vi "Signal Generator.vi"() -> ()   [LabVIEW 2020]
uses:
  <userlib>/ArtDAQ/_SubVI/ArtDAQ_CreateAOVoltageChan.vi
  <vilib>/Utility/xml.llb/Read From XML File(string).vi
  <vilib>/Utility/config.llb/Read Key (I32).vi
  <vilib>/Utility/config.llb/Read Key (Double).vi
  <vilib>/Utility/config.llb/Read Key (Boolean).vi
  <userlib>/ArtDAQ/_SubVI/ArtDAQ_Write Analog DBL NChan NSamp.vi
  <userlib>/ArtDAQ/_SubVI/ArtDAQ_CfgSampClkTiming.vi
  <vilib>/Utility/xml.llb/Write to XML File(string).vi
  <vilib>/Utility/config.llb/Write Key (U32).vi
  <vilib>/Utility/config.llb/Write Key (Double).vi
  <vilib>/Utility/config.llb/Write Key (Boolean).vi
  <vilib>/measure/NI_MABase.lvlib
  <vilib>/Utility/config.llb/NI_LVConfig.lvlib
  Parameter Settings.vi
panel:
  out "车型数组":string[](array[string])
  in  "Stop":bool
  in  "AO3 Channel":u32(ring)=4 items=["Hall Channel 1", "Hall Channel 2", "ME Channel 1", "ME Channel 2", "ME Channel 3", "ME Channel 4"]
  in  "AO2 Channel":u32(ring)=3 items=["Hall Channel 1", "Hall Channel 1", "ME Channel 1", "ME Channel 2", "ME Channel 3", "ME Channel 4"]
  in  "AO1 Channel":u32(ring)=2 items=["Hall Channel 1", "Hall Channel 2", "ME Channel 1", "ME Channel 2", "ME Channel 3", "ME Channel 4"]
  in  "AO0 Channel":u32(ring) items=["Hall Channel 1", "Hall Channel 2", "ME Channel 1", "ME Channel 2", "ME Channel 3", "ME Channel 3"]
  out "转速表":dbl(knob) scale=0.0..3000.0
  in  "Speed FM":dbl(knob)=583.5936811226446 caption="转速调频" scale=50.0..1000.0
  in  "Brand":u32(ring)=2 items=["Carter", "Keith", "Hitachi", "Kobelco", "Volvo", "Modern", "Komatsu", "Sumitomo"]
  in  "Vehicle Signal":u32(ring) items=["58+2 sinusoid SK140-8", "Hino J05E new 4 cylinder", "Hino J08E new 6 cylinder"]
  out "ME Channel 4":waveform(dbl)(graph)
  out "ME Channel 3":dynamicdata(graph)
  out "ME Channel 2":waveform(dbl)(graph)
  out "ME Channel 1":dynamicdata(graph)
  out "Hall Channel 2":waveform(dbl)(graph)
  out "Hall Channel 1":T1
  out "数组大小":i32
  out "品牌":string
  out "品牌数组":string[](array[string])
  in  "error":errorcluster caption="错误输入（无错误）"
  in  "字符串数组类型":string[](array[string])
  out "数值合法":bool
  out "凸轮轴参数":T2
  out "0凸轮轴信号类型":u32
  out "0凸轮轴电压幅值":dbl format="%#.1f"
  out "0信号个数":dbl=7.0 caption="信号个数" format="%#.1f"
  out "0凸轮轴个数":dbl=1.0 caption="凸轮轴个数" format="%#.1f"
  out "0凸轮轴是否取反":bool
  out "0凸轮轴周期":dbl=3.0 caption="凸轮轴周期" format="%#.1f"
  out "0起始偏移":dbl=3.0 caption="凸轮轴周期" format="%#.1f"
  out "0插齿间隔":dbl=3.0 caption="凸轮轴周期" format="%#.1f"
  out "0间隔齿数":dbl=3.0 caption="凸轮轴周期" format="%#.1f"
  out "曲轴参数":T3
  out "0曲轴轴信号类型":u32
  out "0曲轴电压幅值":dbl format="%#.1f"
  out "0总齿数":dbl=7.0 caption="信号个数" format="%#.1f"
  out "0曲轴个数":dbl=1.0 caption="凸轮轴个数" format="%#.1f"
  out "0曲轴是否取反":bool
  out "0缺齿数":dbl=3.0 caption="凸轮轴周期" format="%#.1f"
  out "0曲轴圈数":dbl=3.0 caption="凸轮轴周期" format="%#.1f"
  out "0缺齿偏移":dbl=3.0 caption="凸轮轴周期" format="%#.1f"
  out "品牌车型数组":string[](array[string])
  out "凸轮轴信号类型":u16(ring) items=["磁电式", "霍尔式", "无曲轴"]
  out "每通道采样数":i32
  in  "采样速率":dbl=50000.0
  in  "物理通道":string(combo)="Dev1/ao0:3"
  out "错误输出":errorcluster
  out "曲轴圈数信号":dynamicdata(graph)
  out "1缺齿偏移":dbl=4.0
  out "缺齿偏移":dbl=8.2 format="%_2f"
  out "长平组信号正弦":dynamicdata(graph)
  out "间隔长平+正弦信号":dynamicdata(graph)
  out "曲轴组合波形":waveform(dbl)(graph)
  out "1曲轴圈数":dbl=4.0
  out "曲轴圈数":dbl=8.2
  out "长平组信号":dynamicdata(graph)
  out "间隔长平+凸信号":dynamicdata(graph)
  out "间隔齿数":dbl=3.0
  out "1间隔齿数":dbl=3.0 caption="凸轮轴周期"
  out "1插齿间隔":dbl=3.0 caption="凸轮轴周期"
  out "1起始偏移":dbl=3.0 caption="凸轮轴周期"
  out "插齿间隔":dbl=8.2
  out "起始偏移":dbl=8.2
  out "车型数组大小":i32
  in  "error":errorcluster caption="错误输入（无错误）"
  in  "字符串数组类型":string[](array[string])
  out "凸轮轴周期·":dbl=8.2 caption="凸轮轴周期"
  out "凸轮轴个数":dbl=8.2
  out "曲轴个数":dbl=8.2
  out "信号个数":dbl=8.2
  out "凸轮轴是否取反":bool
  out "凸轮轴电压幅值":dbl=8.2 format="%0.2p"
  out "曲轴是否取反":bool
  out "曲轴信号类型":u16(ring) items=["磁电式", "霍尔式", "无曲轴"]
  out "缺齿数":dbl=4.0
  out "总齿数":dbl=60.0
  out "曲轴电压幅值":dbl=8.2 format="%0.2p"
  out "1凸轮轴周期·":dbl=3.0 caption="凸轮轴周期"
  out "1凸轮轴是否取反":bool
  out "1凸轮轴个数":dbl=1.0 caption="凸轮轴个数"
  out "1信号个数":dbl=7.0 caption="信号个数"
  out "1凸轮轴电压幅值":dbl=5.0 caption="凸轮轴电压幅值" format="%0.2p"
  out "1凸轮轴信号类型":u16(ring)=1 items=["磁电式", "霍尔式", "无凸轮轴"]
  out "1缺齿数":dbl=4.0
  out "1总齿数":dbl=60.0
  out "1曲轴个数":dbl=2.0 caption="曲轴个数"
  out "1曲轴是否取反":bool
  out "1曲轴电压幅值":dbl=18.0 caption="曲轴电压幅值" format="%0.2p"
  out "1曲轴信号类型":u16(ring) items=["磁电式", "霍尔式", "无曲轴"]
  out "1波形图":waveform(dbl)(graph)
  out "起始偏移（方波）":dbl
  out "起始偏移（正弦）":dbl=0.5
  out "中短平+2正弦":dynamicdata(graph)
  out "长平+1正弦":dynamicdata(graph)
  out "长水平线数量（正弦）":dbl
  out "一个正弦波形图":waveform(dbl)(graph)
  out "起始水平线个数（正弦）":dbl
  out "起始平+1正弦":dynamicdata(graph)
  out "6波形图":waveform(dbl)(graph)
  out "5波形图":waveform(dbl)(graph)
  out "起始水平线个数（方波）":dbl
  out "长平+1凸":dynamicdata(graph)
  out "长水平线数量（方波）":dbl
  out "曲轴":dynamicdata(graph)
  out "曲轴方波缺齿波形图":dynamicdata(graph)
  out "曲轴方波偏移量":dbl=8.2 format="%0.2p"
  out "曲轴方波波形图":waveform(dbl)(graph)
  out "中、短平+2凸":dynamicdata(graph)
  out "起始平+1凸":dynamicdata(graph)
  out "一个凸起波形图":dynamicdata(graph)
  out "曲轴正弦偏移量":dbl caption="偏移量" format="%0.2p"
  out "曲轴正弦波形图":waveform(dbl)(graph)
  out "完\n整\n缺\n齿\n波":waveform(dbl)(graph)
  out "未\n翻\n转\n半\n缺\n齿":dynamicdata(graph)
  out "圆\n弧\n+\n水\n平":dynamicdata(graph)
  out "半\n缺\n齿\n水\n平\n线":waveform(dbl)(graph)
  out "圆\n弧":waveform(dbl)(graph)
  out "t0":timestamp
  out "x轴取点间隔":dbl
  out "循环次数":i32
  out "圆弧点数":dbl=33.0 format="%0.2p"
  out "dt":dbl
  out "圆半径":dbl=2.48 format="%0.2p"
  out "部分\n正弦\n波形图":waveform(dbl)(graph)
  in  "波形发生率Fs":dbl=50000.0
types:
  T1 = typedef "控件 1.ctl" = waveform(dbl)
  T2 = cluster{"0凸轮轴信号类型":u32, "0凸轮轴电压幅值":dbl, "0信号个数":dbl, "0凸轮轴个数":dbl, "0凸轮轴是否取反":bool, "0凸轮轴周期":dbl, "0起始偏移":dbl, "0插齿间隔":dbl, "0间隔齿数":dbl}
  T3 = cluster{"0曲轴轴信号类型":u32, "0曲轴电压幅值":dbl, "0总齿数":dbl, "0曲轴个数":dbl, "0曲轴是否取反":bool, "0却齿数":dbl, "0曲轴圈数":dbl, "0缺齿偏移":dbl}
  T4 = typedef "NI_LVConfig.lvlib/Config Data RefNum.ctl" = refnum<k1>
  T5 = cluster{"0曲轴轴信号类型":u32, "0曲轴电压幅值":dbl, "0总齿数":dbl, "0曲轴个数":dbl, "0曲轴是否取反":bool, "0缺齿数":dbl, "0曲轴圈数":dbl, "0缺齿偏移":dbl}
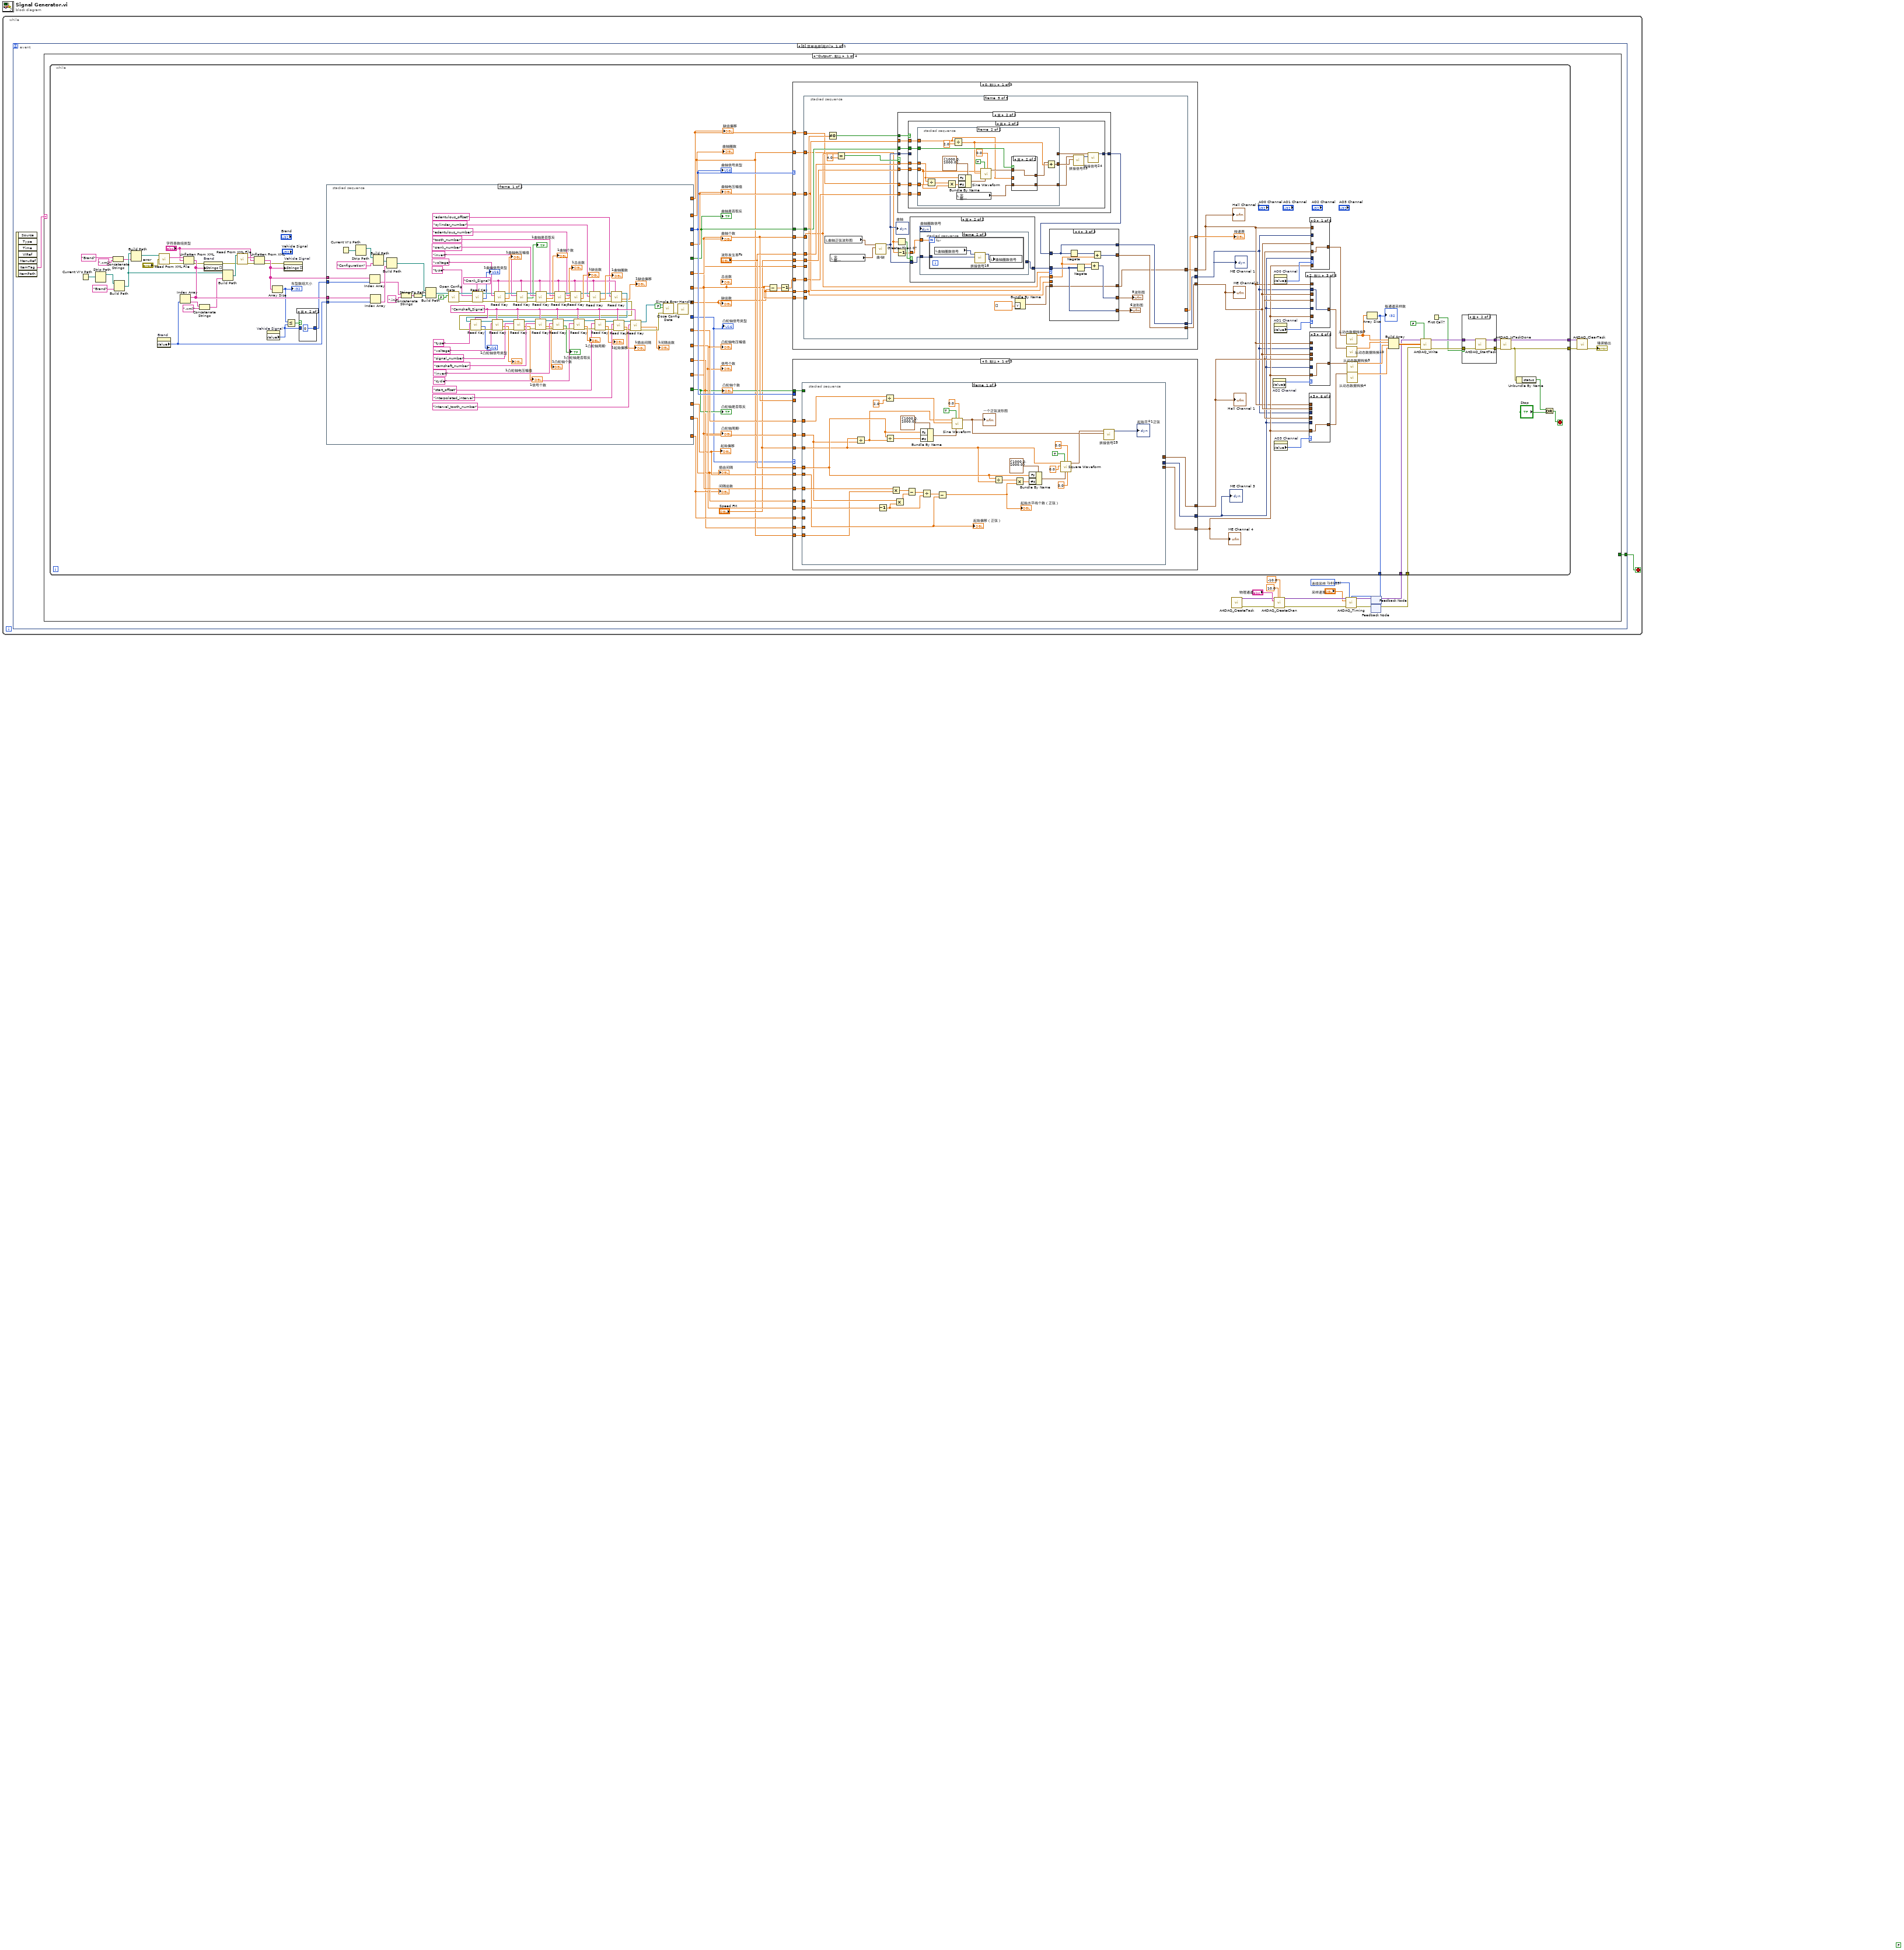
[diagram p0: block diagram]
diagram:
  (unwired) FALSE
  n1 = while {
    stop <- w1 stop-if-true
    n2 = event shown="[0] 菜单选择(用户)" {
      selector: _ -> [_]
      dyn-events: _ -> [_]
      timeout: _ -> [_]
      tunnel: [w3] -> w1
      event Menu Selection (User) {
        n3 = event-data() -> ("ItemTag"=w2:string)  [unwired: 1 in, 6 out]
        n4 = case shown="\"Output\", 默认" w2 {
          selector: w2 -> [_ _ _ w1225]
          tunnel: [_ TRUE _ _] -> w3
          frame "Output", Default {
            w13 = 10123 items=["有限点采样"=10178, "连续采样"=10123] ("SampleMode")
            n5 = call <userlib>:"ArtDAQ_CreateTask.vi"() -> ("任务句柄"=w14:variant, "错误输出"=w15:errorcluster)  [unwired: 14 in]
            n6 = call-poly <userlib>:"ArtDAQ_CreateChan.vi"("任务句柄"=w14, "最大值"=10.0, "最小值"=-10.0, "物理通道"="物理通道", "错误输入"=w15) -> ("任务句柄"=w18:variant, "错误输出"=w19:errorcluster)  [unwired: 9 in]
            n7 = feedback #1() -> (w7:errorcluster)  [unwired: 1 in]
            n8 = feedback #2() -> (w8:variant)  [unwired: 1 in]
            n9 = while {
              tunnel: [w31] -> w6
              tunnel: w8 -> [w21]
              tunnel: w7 -> [w28]
              tunnel: [w23] -> w5
              tunnel: [w22] -> w4
              stop <- w32 stop-if-true
              n10 = Current VI's Path() -> (path=w82:path)
              n11 = Strip Path(path=w82) -> (stripped path=w81:path)  [unwired: 1 out]
              n12 = Concatenate Strings("Brand" ("字符串"), ".xml") -> (w72:string)
              n13 = Build Path(base path=w81, name or relative path="Brand" ("名称或相对路径")) -> (appended path=w73:path)
              n14 = Build Path(base path=w73, name or relative path=w72) -> (appended path=w71:path)
              n15 = property on="Brand" class="Ring (严格)"() -> ("Value"=w88:u32)  [unwired: 2 in, 2 out]
              n16 = call-poly <vilib>:"Read From XML File.vi"("error in (no error)"="error", "XML File Path"=w71) -> ("error out"=w85:errorcluster, "XML Elements"=w84:string)  [unwired: 7 in, 1 out]
              n17 = Unflatten From XML(xml string=w84, type="字符串数组类型", error in (no error)=w85) -> (value=w89:string[], error out=w77:errorcluster)
              n18 = Index Array(array=w89, index=w88) -> (element=w83:string)
              n19 = Concatenate Strings(w83, ".xml") -> (w80:string)
              n20 = property on="Brand" class="Ring (严格)"(error in=w77, "Strings []"=w89) -> (error out=w30:errorcluster)  [unwired: 1 in, 1 out]
              n21 = Build Path(base path=w73, name or relative path=w80) -> (appended path=w66:path)
              n22 = call-poly <vilib>:"Read From XML File.vi"("error in (no error)"=w30, "XML File Path"=w66) -> ("error out"=w70:errorcluster, "XML Elements"=w69:string)  [unwired: 7 in, 1 out]
              n23 = Unflatten From XML(xml string=w69, type="字符串数组类型", error in (no error)=w70) -> (value=w87:string[], error out=w68:errorcluster)
              n24 = property on="Vehicle Signal" class="Ring (严格)"() -> ("Value"=w64:u32)  [unwired: 2 in, 2 out]
              n25 = Array Size(array=w87) -> (size(s)=w63:i32)
              "车型数组大小" <- w63
              n26 = property on="Vehicle Signal" class="Ring (严格)"(error in=w68, "Strings []"=w87) -> ()  [unwired: 1 in, 2 out]
              n27 = Less Or Equal?(x=w63, y=w64) -> (x <= y?=w65:bool)
              n28 = case shown="真" w65 {
                tunnel: w64 -> [w134 _]
                tunnel: [w134 0] -> w86
                frame False {
                }
                frame True {
                }
              }
              n29 = stacked-sequence {
                tunnel: [_ w242] -> w99
                tunnel: [_ w241] -> w98
                tunnel: [_ w240] -> w97
                tunnel: [_ w239] -> w96
                tunnel: [_ w238] -> w95
                tunnel: [_ w237] -> w94
                tunnel: [_ w236] -> w44
                tunnel: [_ w235] -> w93
                tunnel: [_ w234] -> w92
                tunnel: [_ w233] -> w24
                tunnel: [_ w232] -> w91
                tunnel: [_ w231] -> w90
                tunnel: w89 -> [w170 _]
                tunnel: w87 -> [w167 _]
                tunnel: w88 -> [w163 _]
                tunnel: w86 -> [w162 _]
                tunnel: [_ w230] -> w62
                tunnel: [_ w229] -> w61
                tunnel: [_ w228] -> w60
                tunnel: [_ w227] -> w25
                tunnel: [_ w226] -> w59
                frame #0 {
                  w149 = "Camshaft_Signal" ("section")
                  w139 = "Crank_Signal" ("section")
                  n30 = Current VI's Path() -> (path=w176:path)
                  n31 = Strip Path(path=w176) -> (stripped path=w175:path)  [unwired: 1 out]
                  n32 = Index Array(array=w167, index=w162) -> (element=w166:string)
                  n33 = Index Array(array=w170, index=w163) -> (element=w169:string)
                  n34 = Build Path(base path=w175, name or relative path="Configuration" ("名称或相对路径")) -> (appended path=w171:path)
                  n35 = Build Path(base path=w171, name or relative path=w169) -> (appended path=w172:path)
                  n36 = Concatenate Strings(w166, ".ini" ("字符串")) -> (w164:string)
                  n37 = String To Path(string=w164) -> (path=w165:path)
                  n38 = Build Path(base path=w172, name or relative path=w165) -> (appended path=w173:path)
                  n39 = call <vilib>:"Open Config Data.vi"("create file if necessary (T)"=FALSE ("create file if necessary? (T)"), "configuration file path"=w173) -> ("error out"=w205:errorcluster, "refnum"=w203:T4)  [unwired: 7 in, 1 out]
                  n40 = call-poly <vilib>:"Read Key.vi"("section"=w139, "error in (no error)"=w205, "key"="type", "refnum"=w203) -> ("error out"=w206:errorcluster, "value"=→"1曲轴信号类型":i32, "refnum out"=w204:T4)  [unwired: 1 in, 4 out]
                  n41 = call-poly <vilib>:"Read Key.vi"("section"=w139, "error in (no error)"=w206, "key"="voltage" ("键2"), "refnum"=w204) -> ("error out"=w201:errorcluster, "value"=→"1曲轴电压幅值":dbl, "refnum out"=w200:T4)  [unwired: 1 in, 4 out]
                  n42 = call-poly <vilib>:"Read Key.vi"("section"=w139, "error in (no error)"=w201, "key"="invert" ("键3"), "refnum"=w200) -> ("error out"=w198:errorcluster, "value"=→"1曲轴是否取反":bool, "refnum out"=w197:T4)  [unwired: 1 in, 4 out]
                  n43 = call-poly <vilib>:"Read Key.vi"("section"=w139, "error in (no error)"=w198, "key"="crank_number" ("键3"), "refnum"=w197) -> ("error out"=w195:errorcluster, "value"=→"1曲轴个数":dbl, "refnum out"=w194:T4)  [unwired: 1 in, 4 out]
                  n44 = call-poly <vilib>:"Read Key.vi"("section"=w139, "error in (no error)"=w195, "key"="tooth_number" ("键3"), "refnum"=w194) -> ("error out"=w192:errorcluster, "value"=→"1总齿数":dbl, "refnum out"=w193:T4)  [unwired: 1 in, 4 out]
                  n45 = call-poly <vilib>:"Read Key.vi"("section"=w139, "error in (no error)"=w192, "key"="edentulous_number" ("键3"), "refnum"=w193) -> ("error out"=w145:errorcluster, "value"=→"1缺齿数":dbl, "refnum out"=w144:T4)  [unwired: 1 in, 4 out]
                  n46 = call-poly <vilib>:"Read Key.vi"("section"=w139, "error in (no error)"=w145, "key"="cylinder_number" ("键3"), "refnum"=w144) -> ("error out"=w138:errorcluster, "value"=→"1曲轴圈数":dbl, "refnum out"=w141:T4)  [unwired: 1 in, 4 out]
                  n47 = call-poly <vilib>:"Read Key.vi"("section"=w139, "error in (no error)"=w138, "key"="edentulous_offset" ("键2"), "refnum"=w141) -> ("error out"=w137:errorcluster, "value"=→"1缺齿偏移":dbl, "refnum out"=w142:T4)  [unwired: 1 in, 4 out]
                  n48 = call-poly <vilib>:"Read Key.vi"("section"=w149, "error in (no error)"=w137, "key"="type" ("键3"), "refnum"=w142) -> ("error out"=w225:errorcluster, "value"=→"1凸轮轴信号类型":i32, "refnum out"=w224:T4)  [unwired: 2 in, 3 out]
                  n49 = call-poly <vilib>:"Read Key.vi"("section"=w149, "error in (no error)"=w225, "key"="voltage" ("键3"), "refnum"=w224) -> ("error out"=w218:errorcluster, "value"=→"1凸轮轴电压幅值":dbl, "refnum out"=w216:T4)  [unwired: 2 in, 3 out]
                  n50 = call-poly <vilib>:"Read Key.vi"("section"=w149, "error in (no error)"=w218, "key"="signal_number" ("键3"), "refnum"=w216) -> ("error out"=w181:errorcluster, "value"=→"1信号个数":dbl, "refnum out"=w215:T4)  [unwired: 2 in, 3 out]
                  n51 = call-poly <vilib>:"Read Key.vi"("section"=w149, "error in (no error)"=w181, "key"="camshaft_number" ("键3"), "refnum"=w215) -> ("error out"=w217:errorcluster, "value"=→"1凸轮轴个数":dbl, "refnum out"=w214:T4)  [unwired: 2 in, 3 out]
                  n52 = call-poly <vilib>:"Read Key.vi"("section"=w149, "error in (no error)"=w217, "key"="invert" ("键2"), "refnum"=w214) -> ("error out"=w219:errorcluster, "value"=→"1凸轮轴是否取反":bool, "refnum out"=w213:T4)  [unwired: 2 in, 3 out]
                  n53 = call-poly <vilib>:"Read Key.vi"("section"=w149, "error in (no error)"=w219, "key"="cycle", "refnum"=w213) -> ("error out"=w158:errorcluster, "value"=→"1凸轮轴周期·":dbl, "refnum out"=w161:T4)  [unwired: 2 in, 3 out]
                  n54 = call-poly <vilib>:"Read Key.vi"("section"=w149, "error in (no error)"=w158, "key"="start_offset" ("键2"), "refnum"=w161) -> ("error out"=w159:errorcluster, "value"=→"1起始偏移":dbl, "refnum out"=w160:T4)  [unwired: 2 in, 3 out]
                  n55 = call-poly <vilib>:"Read Key.vi"("section"=w149, "error in (no error)"=w159, "key"="interpolated_interval", "refnum"=w160) -> ("error out"=w152:errorcluster, "value"=→"1插齿间隔":dbl, "refnum out"=w153:T4)  [unwired: 2 in, 3 out]
                  n56 = call-poly <vilib>:"Read Key.vi"("section"=w149, "error in (no error)"=w152, "key"="interval_tooth_number", "refnum"=w153) -> ("error out"=w151:errorcluster, "value"=→"1间隔齿数":dbl, "refnum out"=w150:T4)  [unwired: 2 in, 3 out]
                  n57 = call <vilib>:"Close Config Data.vi"("error in (no error)"=w151, "write file if changed (T)"=FALSE ("write configuration file? (T)"), "refnum"=w150) -> ("error out"=w220:errorcluster)  [unwired: 8 out]
                  n58 = call <vilib>:"Simple Error Handler.vi"("error in (no error)"=w220) -> ()  [unwired: 1 in, 8 out]
                }
                frame #1 {
                  n59 = local read "1缺齿偏移"() -> (w226:dbl)
                  n60 = local read "1曲轴圈数"() -> (w227:dbl)
                  n61 = local read "1曲轴信号类型"() -> (w242:u16)
                  n62 = local read "1曲轴电压幅值"() -> (w241:dbl)
                  n63 = local read "1曲轴是否取反"() -> (w240:bool)
                  n64 = local read "1曲轴个数"() -> (w239:dbl)
                  n65 = local read "1总齿数"() -> (w238:dbl)
                  n66 = local read "1缺齿数"() -> (w237:dbl)
                  n67 = local read "1凸轮轴信号类型"() -> (w236:u16)
                  n68 = local read "1凸轮轴电压幅值"() -> (w235:dbl)
                  n69 = local read "1信号个数"() -> (w234:dbl)
                  n70 = local read "1凸轮轴个数"() -> (w233:dbl)
                  n71 = local read "1凸轮轴周期·"() -> (w231:dbl)
                  n72 = local read "1凸轮轴是否取反"() -> (w232:bool)
                  n73 = local read "1起始偏移"() -> (w230:dbl)
                  n74 = local read "1插齿间隔"() -> (w229:dbl)
                  n75 = local read "1间隔齿数"() -> (w228:dbl)
                }
              }
              "总齿数" <- w95
              "缺齿数" <- w94
              "曲轴信号类型" <- w99
              "曲轴电压幅值" <- w98
              "曲轴是否取反" <- w97
              "凸轮轴电压幅值" <- w93
              "凸轮轴是否取反" <- w91
              "信号个数" <- w92
              "曲轴个数" <- w96
              "凸轮轴个数" <- w24
              "凸轮轴周期·" <- w90
              "起始偏移" <- w62
              "插齿间隔" <- w61
              "间隔齿数" <- w60
              "曲轴圈数" <- w25
              "缺齿偏移" <- w59
              "凸轮轴信号类型" <- w44
              n76 = Subtract(x=w95, y=w94) -> (x-y=w102:dbl)
              n77 = Decrement(x=w102) -> (x-1=w101:dbl)
              n78 = case shown="0, 默认" w44 {
                tunnel: "Speed FM" -> [w256 w434 _]
                tunnel: "波形发生率Fs" -> [w255 w433 _]
                tunnel: w95 -> [w254 w432 _]
                tunnel: w93 -> [w257 w431 _]
                tunnel: [w248 w430 w680] -> w42
                tunnel: w92 -> [w253 w429 _]
                tunnel: [w249 w428 w677] -> w41
                tunnel: [w250 w427 w676] -> w29
                tunnel: w90 -> [w252 w423 _]
                tunnel: w24 -> [w251 w426 w675]
                tunnel: w99 -> [_ _ w687]
                tunnel: w96 -> [_ _ w672]
                tunnel: w91 -> [w247 w425 _]
                tunnel: w62 -> [w246 w420 _]
                tunnel: w61 -> [w245 w421 _]
                tunnel: w60 -> [w243 w419 _]
                tunnel: w25 -> [w244 _ _]
                frame 0, Default {
                  n79 = stacked-sequence {
                    tunnel: w257 -> [w285 _ _ w363]
                    tunnel: w256 -> [w267 w296 w320 w375]
                    tunnel: w255 -> [w274 w295 w319 w376]
                    tunnel: w254 -> [w282 _ _ _]
                    tunnel: w253 -> [w283 _ _ w348]
                    tunnel: w252 -> [w265 _ w312 _]
                    tunnel: w251 -> [_ _ _ w367]
                    tunnel: [_ _ _ w366] -> w250
                    tunnel: [_ _ _ w364] -> w249
                    tunnel: [_ _ _ w361] -> w248
                    tunnel: w247 -> [_ _ _ w357]
                    tunnel: w246 -> [w260 w291 _ _]
                    tunnel: w245 -> [_ _ w309 _]
                    tunnel: w244 -> [w258 _ _ _]
                    tunnel: w243 -> [_ _ _ w347]
                    frame #0 {
                      n80 = Divide(x=w267, y=w265) -> (x/y=w266:dbl)
                      n81 = Decrement(x=w283) -> (x-1=w259:dbl)
                      n82 = Divide(x=w285, y=2.0) -> (x/y=w273:dbl)
                      n83 = Divide(x=w274, y=w266) -> (x/y=w284:dbl)
                      n84 = Multiply(x=w282, y=w258) -> (x*y=w264:dbl)
                      n85 = Multiply(x=w265, y=w259) -> (x*y=w263:dbl)
                      n86 = Subtract(x=w264, y=w263) -> (x-y=w262:dbl)
                      n87 = Bundle By Name(cluster=cluster{"Fs":dbl, "#s":dbl} {"Fs"=1000.0, "#s"=1000.0} ("sampling info"), "Fs"=w274, "#s"=w284) -> (w289:cluster{"Fs":dbl, "#s":dbl})
                      n88 = Divide(x=w262, y=w259) -> (x/y=w261:dbl)
                      n89 = Subtract(x=w261, y=w260) -> (x-y=w275:dbl)
                      "起始水平线个数（正弦）" <- w275
                      n90 = call <vilib>:"Sine Waveform.vi"("offset"=0.0, "sampling info"=w289, "reset signal"=TRUE, "amplitude"=w273, "frequency"=w266) -> ("signal out"=w268:waveform(dbl))  [unwired: 5 in, 1 out]
                      "一个正弦波形图" <- w268
                      n91 = Divide(x=w274, y=w267) -> (x/y=w279:dbl)
                      n92 = Multiply(x=w279, y=w275) -> (x*y=w278:dbl)
                      n93 = Bundle By Name(cluster=cluster{"Fs":dbl, "#s":dbl} {"Fs"=1000.0, "#s"=1000.0} ("sampling info"), "Fs"=w274, "#s"=w278) -> (w280:cluster{"Fs":dbl, "#s":dbl})
                      n94 = call <vilib>:"Square Waveform.vi"("duty cycle (%)"=0.0, "offset"=0.0, "sampling info"=w280, "reset signal"=TRUE, "amplitude"=0.0, "frequency"=w267) -> ("signal out"=w271:waveform(dbl))  [unwired: 4 in, 1 out]
                      n95 = call "拼接信号25"("Input Signal B"=w268, "Input Signal A"=w271) -> ("Appended Signals"=→"起始平+1正弦":dynamicdata)  [unwired: 8 in, 1 out]
                      "起始偏移（正弦）" <- w260
                    }
                    frame #1 {
                      n96 = local read "起始水平线个数（正弦）"() -> (w306:dbl)
                      n97 = Divide(x=w295, y=w296) -> (x/y=w303:dbl)
                      n98 = Add(x=w306, y=w291) -> (x+y=w297:dbl)
                      "长水平线数量（正弦）" <- w297
                      n99 = Multiply(x=w303, y=w297) -> (x*y=w302:dbl)
                      n100 = Bundle By Name(cluster=cluster{"Fs":dbl, "#s":dbl} {"Fs"=1000.0, "#s"=1000.0} ("sampling info"), "Fs"=w295, "#s"=w302) -> (w304:cluster{"Fs":dbl, "#s":dbl})
                      n101 = call <vilib>:"Square Waveform.vi"("duty cycle (%)"=0.0, "offset"=0.0, "sampling info"=w304, "reset signal"=TRUE, "amplitude"=0.0, "frequency"=w296) -> ("signal out"=w294:waveform(dbl))  [unwired: 4 in, 1 out]
                      n102 = local read "一个正弦波形图"() -> (w293:waveform(dbl))
                      n103 = call "拼接信号26"("Input Signal B"=w293, "Input Signal A"=w294) -> ("Appended Signals"=→"长平+1正弦":dynamicdata)  [unwired: 8 in, 1 out]
                    }
                    frame #2 {
                      n104 = local read "长水平线数量（正弦）"() -> (w318:dbl)
                      n105 = local read "一个正弦波形图"() -> (w308:waveform(dbl))
                      n106 = Equal To 0?(x=w309) -> (x = 0?=w310:bool)
                      n107 = Subtract(x=w318, y=w312) -> (x-y=w311:dbl)
                      n108 = case shown="假" w310 {
                        tunnel: w320 -> [_ w335]
                        tunnel: w319 -> [_ w334]
                        tunnel: w309 -> [_ w333]
                        tunnel: w308 -> [w329 w332]
                        tunnel: [w329 w330] -> w307
                        frame True {
                        }
                        frame False {
                          n109 = Divide(x=w334, y=w335) -> (x/y=w341:dbl)
                          n110 = Multiply(x=w341, y=w333) -> (x*y=w340:dbl)
                          n111 = Bundle By Name(cluster=cluster{"Fs":dbl, "#s":dbl} {"Fs"=1000.0, "#s"=1000.0} ("sampling info"), "Fs"=w334, "#s"=w340) -> (w342:cluster{"Fs":dbl, "#s":dbl})
                          n112 = call <vilib>:"Square Waveform.vi"("duty cycle (%)"=0.0, "offset"=0.0, "sampling info"=w342, "reset signal"=TRUE, "amplitude"=0.0, "frequency"=w335) -> ("signal out"=w331:waveform(dbl))  [unwired: 4 in, 1 out]
                          n113 = call "拼接信号28"("Input Signal B"=w332, "Input Signal A"=w331) -> ("Appended Signals"=w330:dynamicdata)  [unwired: 8 in, 1 out]
                        }
                      }
                      n114 = Divide(x=w319, y=w320) -> (x/y=w326:dbl)
                      n115 = Subtract(x=w311, y=w309) -> (x-y=w317:dbl)
                      n116 = Multiply(x=w326, y=w317) -> (x*y=w325:dbl)
                      n117 = Bundle By Name(cluster=cluster{"Fs":dbl, "#s":dbl} {"Fs"=1000.0, "#s"=1000.0} ("sampling info"), "Fs"=w319, "#s"=w325) -> (w327:cluster{"Fs":dbl, "#s":dbl})
                      n118 = call <vilib>:"Square Waveform.vi"("duty cycle (%)"=0.0, "offset"=0.0, "sampling info"=w327, "reset signal"=TRUE, "amplitude"=0.0, "frequency"=w320) -> ("signal out"=w315:waveform(dbl))  [unwired: 4 in, 1 out]
                      n119 = local read "一个正弦波形图"() -> (w316:waveform(dbl))
                      n120 = call "拼接信号27"("Input Signal B"=w316, "Input Signal A"=w315) -> ("Appended Signals"=w314:dynamicdata)  [unwired: 8 in, 1 out]
                      n121 = call "拼接信号29"("Input Signal B"=w307, "Input Signal A"=w314) -> ("Appended Signals"=→"中短平+2正弦":dynamicdata)  [unwired: 8 in, 1 out]
                    }
                    frame #3 {
                      n122 = local read "起始偏移（正弦）"() -> (w368:dbl)
                      n123 = Greater Or Equal?(x=w347, y=2.0) -> (x >= y?=w344:bool)
                      n124 = case shown="真" w344 {
                        tunnel: [w394 w399] -> w346
                        tunnel: w347 -> [w393 w398]
                        frame False {
                          n125 = case shown="1, 默认" w393 {
                            tunnel: [w395] -> w394
                            frame 1, Default {
                              n126 = local read "中短平+2正弦"() -> (w396:dynamicdata)
                              n127 = local read "起始平+1正弦"() -> (w397:dynamicdata)
                              n128 = call "拼接信号19"("Input Signal B"=w396, "Input Signal A"=w397) -> ("Appended Signals"=w395:dynamicdata)  [unwired: 8 in, 1 out]
                            }
                          }
                        }
                        frame True {
                          n129 = stacked-sequence {
                            tunnel: [_ _ w408] -> w399
                            tunnel: w398 -> [_ w402 _]
                            frame #0 {
                              n130 = local read "起始平+1正弦"() -> (w400:dynamicdata)
                              n131 = local write "间隔长平+正弦信号"(w400) -> ()
                            }
                            frame #1 {
                              n132 = Decrement(x=w402) -> (x-1=w401:dbl)
                              n133 = for {
                                N: w401 -> [_]
                                n134 = local read "间隔长平+正弦信号"() -> (w405:dynamicdata)
                                n135 = local read "长平+1正弦"() -> (w404:dynamicdata)
                                n136 = call "拼接信号30"("Input Signal B"=w404, "Input Signal A"=w405) -> ("Appended Signals"=w403:dynamicdata)  [unwired: 8 in, 1 out]
                                n137 = local write "间隔长平+正弦信号"(w403) -> ()
                              }
                            }
                            frame #2 {
                              n138 = local read "间隔长平+正弦信号"() -> (w407:dynamicdata)
                              n139 = local read "中短平+2正弦"() -> (w406:dynamicdata)
                              n140 = call "拼接信号31"("Input Signal B"=w406, "Input Signal A"=w407) -> ("Appended Signals"=w408:dynamicdata)  [unwired: 8 in, 1 out]
                            }
                          }
                        }
                      }
                      n141 = Divide(x=w376, y=w375) -> (x/y=w382:dbl)
                      n142 = Multiply(x=w382, y=w368) -> (x*y=w381:dbl)
                      n143 = Bundle By Name(cluster=cluster{"Fs":dbl, "#s":dbl} {"Fs"=1000.0, "#s"=1000.0} ("sampling info"), "Fs"=w376, "#s"=w381) -> (w383:cluster{"Fs":dbl, "#s":dbl})
                      n144 = call <vilib>:"Square Waveform.vi"("duty cycle (%)"=0.0, "offset"=0.0, "sampling info"=w383, "reset signal"=TRUE, "amplitude"=0.0, "frequency"=w375) -> ("signal out"=w369:waveform(dbl))  [unwired: 4 in, 1 out]
                      n145 = local read "长平+1正弦"() -> (w370:dynamicdata)
                      n146 = Subtract(x=w348, y=4.0) -> (x-y=w354:dbl)
                      n147 = Decrement(x=w347) -> (x-1=w353:dbl)
                      n148 = Subtract(x=w354, y=w353) -> (x-y=w351:dbl)
                      n149 = Greater Or Equal?(x=w351, y=1.0) -> (x >= y?=w350:bool)
                      n150 = Decrement(x=w351) -> (x-1=w349:dbl)
                      n151 = call "拼接信号32"("Input Signal B"=w369, "Input Signal A"=w370) -> ("Appended Signals"=w374:dynamicdata)  [unwired: 8 in, 1 out]
                      n152 = case shown="真" w350 {
                        tunnel: w349 -> [_ w386]
                        tunnel: [_ w385] -> w345
                        frame False {
                        }
                        frame True {
                          n153 = stacked-sequence {
                            tunnel: w386 -> [_ w388 _]
                            tunnel: [_ _ w392] -> w385
                            frame #0 {
                              n154 = local read "长平+1正弦"() -> (w387:dynamicdata)
                              n155 = local write "长平组信号正弦"(w387) -> ()
                            }
                            frame #1 {
                              n156 = for {
                                N: w388 -> [_]
                                n157 = local read "长平组信号正弦"() -> (w391:dynamicdata)
                                n158 = local read "长平+1正弦"() -> (w390:dynamicdata)
                                n159 = call "拼接信号33"("Input Signal B"=w390, "Input Signal A"=w391) -> ("Appended Signals"=w389:dynamicdata)  [unwired: 8 in, 1 out]
                                n160 = local write "长平组信号正弦"(w389) -> ()
                              }
                            }
                            frame #2 {
                              n161 = local read "长平组信号正弦"() -> (w392:dynamicdata)
                            }
                          }
                        }
                      }
                      n162 = call "拼接信号34"("Input Signal B"=w345, "Input Signal A"=w346) -> ("Appended Signals"=w373:dynamicdata)  [unwired: 8 in, 1 out]
                      n163 = Bundle By Name("Y"=dbl[] []) -> (w362:waveform(dbl))  [unwired: 1 in]
                      n164 = call "拼接信号35"("Input Signal B"=w374, "Input Signal A"=w373) -> ("Appended Signals"=w360:dynamicdata)  [unwired: 8 in, 1 out]
                      n165 = case shown="真" w357 {
                        tunnel: [w409 w411] -> w359
                        tunnel: w360 -> [w409 w410]
                        frame False {
                        }
                        frame True {
                          n166 = Negate(x=w410) -> (-x=w411:dynamicdata)
                        }
                      }
                      n167 = Divide(x=w363, y=2.0) -> (x/y=w371:dbl)
                      n168 = Add(x=w371, y=w359) -> (x+y=w358:dynamicdata)
                      n169 = case shown="2, 默认" w367 {
                        tunnel: w358 -> [w413 w416]
                        tunnel: [w413 w416] -> w366
                        tunnel: [w412 w417] -> w364
                        tunnel: w363 -> [_ w415]
                        tunnel: w362 -> [w412 w414]
                        tunnel: [w412 w414] -> w361
                        frame 1 {
                        }
                        frame 2, Default {
                          n170 = Negate(x=w416) -> (-x=w418:dynamicdata)
                          n171 = Add(x=w418, y=w415) -> (x+y=w417:dynamicdata)
                        }
                      }
                    }
                  }
                }
                frame 1 {
                  n172 = Not Equal?(x=w423, y=1.0) -> (x != y?=w422:bool)
                  n173 = case shown="真" w422 {
                    tunnel: w434 -> [w443 w487]
                    tunnel: w433 -> [w455 w486]
                    tunnel: w432 -> [_ w485]
                    tunnel: w431 -> [w435 w484]
                    tunnel: [w453 w483] -> w430
                    tunnel: w429 -> [w456 w482]
                    tunnel: [w451 w481] -> w428
                    tunnel: [w451 w480] -> w427
                    tunnel: w426 -> [_ w479]
                    tunnel: w425 -> [w450 w478]
                    tunnel: w423 -> [w439 w477]
                    tunnel: w421 -> [_ w476]
                    tunnel: w420 -> [_ w475]
                    tunnel: w419 -> [_ w474]
                    frame False {
                      n174 = Divide(x=w435, y=2.0) -> (x/y=w436:dbl)
                      n175 = Divide(x=w455, y=w443) -> (x/y=w459:dbl)
                      n176 = Divide(x=w455, y=w443) -> (x/y=w440:dbl)
                      n177 = Multiply(x=w459, y=w456) -> (x*y=w458:dbl)
                      n178 = Bundle By Name(cluster=cluster{"Fs":dbl, "#s":dbl} {"Fs"=1000.0, "#s"=1000.0} ("sampling info"), "Fs"=w455, "#s"=w458) -> (w464:cluster{"Fs":dbl, "#s":dbl})
                      n179 = Multiply(x=w440, y=w439) -> (x*y=w441:dbl)
                      n180 = Bundle By Name(cluster=cluster{"Fs":dbl, "#s":dbl} {"Fs"=1000.0, "#s"=1000.0} ("sampling info"), "Fs"=w455, "#s"=w441) -> (w448:cluster{"Fs":dbl, "#s":dbl})
                      n181 = call <vilib>:"Square Waveform.vi"("duty cycle (%)"=50.0, "offset"=0.0, "sampling info"=w464, "reset signal"=TRUE, "amplitude"=w436, "frequency"=w443) -> ("signal out"=w457:waveform(dbl))  [unwired: 4 in, 1 out]
                      n182 = call <vilib>:"Square Waveform.vi"("duty cycle (%)"=0.0, "offset"=0.0, "sampling info"=w448, "reset signal"=TRUE, "amplitude"=0.0, "frequency"=w443) -> ("signal out"=w444:waveform(dbl))  [unwired: 4 in, 1 out]
                      n183 = case shown="真" w450 {
                        tunnel: w457 -> [w471 w473]
                        tunnel: [w471 w472] -> w438
                        frame False {
                        }
                        frame True {
                          n184 = Negate(x=w473) -> (-x=w472:waveform(dbl))
                        }
                      }
                      n185 = case shown="真" w450 {
                        tunnel: w444 -> [w466 w470]
                        tunnel: [w466 w469] -> w454
                        tunnel: w435 -> [_ w467]
                        frame False {
                        }
                        frame True {
                          n186 = Negate(x=w470) -> (-x=w468:waveform(dbl))
                          n187 = Add(x=w467, y=w468) -> (x+y=w469:waveform(dbl))
                        }
                      }
                      n188 = Add(x=w436, y=w438) -> (x+y=w437:waveform(dbl))
                      n189 = Bundle By Name("Y"=dbl[] []) -> (w451:waveform(dbl))  [unwired: 1 in]
                      n190 = call "拼接信号38"("Input Signal B"=w454, "Input Signal A"=w437) -> ("Appended Signals"=w453:dynamicdata)  [unwired: 8 in, 1 out]
                    }
                    frame True {
                      n191 = stacked-sequence {
                        tunnel: w487 -> [w492 w551 w561 w575 w633]
                        tunnel: w486 -> [w510 w550 w560 w576 w632]
                        tunnel: w485 -> [_ w553 _ _ _]
                        tunnel: w484 -> [w509 w552 w557 w585 w634]
                        tunnel: [_ _ _ _ w623] -> w483
                        tunnel: w482 -> [_ w549 _ _ w611]
                        tunnel: [_ _ _ _ w620] -> w481
                        tunnel: [_ _ _ _ w619] -> w480
                        tunnel: w477 -> [w489 w536 _ w574 _]
                        tunnel: w479 -> [_ _ _ _ w612]
                        tunnel: w478 -> [_ _ _ _ w615]
                        tunnel: w476 -> [_ _ _ w572 _]
                        tunnel: w475 -> [_ w529 w554 _ _]
                        tunnel: w474 -> [_ _ _ _ w608]
                        frame #0 {
                          n192 = Divide(x=w509, y=2.0) -> (x/y=w493:dbl)
                          n193 = Greater?(x=w489, y=2.0) -> (0:w488:bool)
                          n194 = Divide(x=w510, y=w492) -> (x/y=w491:dbl)
                          n195 = case shown="真" w488 {
                            tunnel: w510 -> [_ w524]
                            tunnel: [_ w520] -> w500
                            tunnel: w493 -> [_ w517]
                            tunnel: w492 -> [_ w516]
                            tunnel: w491 -> [_ w514]
                            tunnel: w489 -> [_ w511]
                            frame False {
                            }
                            frame True {
                              n196 = Subtract(x=w511, y=2.0) -> (x-y=w513:dbl)
                              n197 = Multiply(x=w514, y=w513) -> (x*y=w515:dbl)
                              n198 = Bundle By Name(cluster=cluster{"Fs":dbl, "#s":dbl} {"Fs"=1000.0, "#s"=1000.0} ("sampling info"), "Fs"=w524, "#s"=w515) -> (w522:cluster{"Fs":dbl, "#s":dbl})
                              n199 = call <vilib>:"Square Waveform.vi"("duty cycle (%)"=100.0, "offset"=0.0, "sampling info"=w522, "reset signal"=TRUE, "amplitude"=w517, "frequency"=w516) -> ("signal out"=w520:waveform(dbl))  [unwired: 4 in, 1 out]
                            }
                          }
                          n200 = Bundle By Name(cluster=cluster{"Fs":dbl, "#s":dbl} {"Fs"=1000.0, "#s"=1000.0} ("sampling info"), "Fs"=w510, "#s"=w491) -> (w507:cluster{"Fs":dbl, "#s":dbl})
                          n201 = call <vilib>:"Square Waveform.vi"("duty cycle (%)"=50.0, "offset"=0.0, "sampling info"=w507, "reset signal"=TRUE, "amplitude"=w493, "frequency"=w492) -> ("signal out"=w498:waveform(dbl))  [unwired: 4 in, 1 out]
                          n202 = call "从动态数据转换2"("Dynamic Data Type"=w498) -> ("Array"=w505:dbl[])  [unwired: 3 in]
                          n203 = Unbundle By Name(w498) -> ("t0"=w503:timestamp, "dt"=w504:dbl)  [unwired: 1 out]
                          n204 = Reverse 1D Array(array=w505) -> (reversed array=w506:dbl[])
                          n205 = Bundle By Name("Y"=w506, "t0"=w503, "dt"=w504) -> (w501:waveform(dbl))  [unwired: 1 in]
                          n206 = case shown="3, 默认" w489 {
                            tunnel: w501 -> [w527 w528]
                            tunnel: w500 -> [w526 _]
                            tunnel: [w525 w528] -> w499
                            frame 3, Default {
                              n207 = call "拼接信号5"("Input Signal B"=w526, "Input Signal A"=w527) -> ("Appended Signals"=w525:dynamicdata)  [unwired: 8 in, 1 out]
                            }
                            frame 2 {
                            }
                          }
                          n208 = call "拼接信号6"("Input Signal B"=w498, "Input Signal A"=w499) -> ("Appended Signals"=→"一个凸起波形图":dynamicdata)  [unwired: 8 in, 1 out]
                        }
                        frame #1 {
                          n209 = Decrement(x=w549) -> (x-1=w530:dbl)
                          n210 = Multiply(x=w553, y=2.0) -> (x*y=w535:dbl)
                          n211 = Multiply(x=w536, y=w530) -> (x*y=w534:dbl)
                          n212 = Subtract(x=w535, y=w534) -> (x-y=w532:dbl)
                          n213 = Divide(x=w552, y=2.0) -> (x/y=w538:dbl)
                          n214 = Divide(x=w550, y=w551) -> (x/y=w546:dbl)
                          n215 = Divide(x=w532, y=w530) -> (x/y=w531:dbl)
                          n216 = Subtract(x=w531, y=w529) -> (x-y=w540:dbl)
                          "起始水平线个数（方波）" <- w540
                          n217 = Multiply(x=w546, y=w540) -> (x*y=w545:dbl)
                          n218 = Bundle By Name(cluster=cluster{"Fs":dbl, "#s":dbl} {"Fs"=1000.0, "#s"=1000.0} ("sampling info"), "Fs"=w550, "#s"=w545) -> (w547:cluster{"Fs":dbl, "#s":dbl})
                          n219 = call <vilib>:"Square Waveform.vi"("duty cycle (%)"=0.0, "sampling info"=w547, "reset signal"=TRUE, "amplitude"=w538, "frequency"=w551) -> ("signal out"=w544:waveform(dbl))  [unwired: 5 in, 1 out]
                          n220 = local read "一个凸起波形图"() -> (w543:dynamicdata)
                          n221 = call "拼接信号8"("Input Signal B"=w543, "Input Signal A"=w544) -> ("Appended Signals"=→"起始平+1凸":dynamicdata)  [unwired: 8 in, 1 out]
                          "起始偏移（方波）" <- w529
                        }
                        frame #2 {
                          n222 = local read "起始水平线个数（方波）"() -> (w562:dbl)
                          n223 = Divide(x=w557, y=2.0) -> (x/y=w555:dbl)
                          n224 = Add(x=w554, y=w562) -> (x+y=w563:dbl)
                          "长水平线数量（方波）" <- w563
                          n225 = Divide(x=w560, y=w561) -> (x/y=w569:dbl)
                          n226 = Multiply(x=w569, y=w563) -> (x*y=w568:dbl)
                          n227 = Bundle By Name(cluster=cluster{"Fs":dbl, "#s":dbl} {"Fs"=1000.0, "#s"=1000.0} ("sampling info"), "Fs"=w560, "#s"=w568) -> (w570:cluster{"Fs":dbl, "#s":dbl})
                          n228 = local read "一个凸起波形图"() -> (w564:dynamicdata)
                          n229 = call <vilib>:"Square Waveform.vi"("duty cycle (%)"=0.0, "offset"=0.0, "sampling info"=w570, "reset signal"=TRUE, "amplitude"=w555, "frequency"=w561) -> ("signal out"=w565:waveform(dbl))  [unwired: 4 in, 1 out]
                          n230 = call "拼接信号22"("Input Signal B"=w564, "Input Signal A"=w565) -> ("Appended Signals"=→"长平+1凸":dynamicdata)  [unwired: 8 in, 1 out]
                        }
                        frame #3 {
                          n231 = local read "长水平线数量（方波）"() -> (w578:dbl)
                          n232 = Divide(x=w585, y=2.0) -> (x/y=w584:dbl)
                          n233 = Subtract(x=w578, y=w574) -> (x-y=w573:dbl)
                          n234 = Subtract(x=w573, y=w572) -> (x-y=w593:dbl)
                          n235 = Divide(x=w576, y=w575) -> (x/y=w577:dbl)
                          n236 = Multiply(x=w577, y=w593) -> (x*y=w598:dbl)
                          n237 = Multiply(x=w577, y=w572) -> (x*y=w589:dbl)
                          n238 = Bundle By Name(cluster=cluster{"Fs":dbl, "#s":dbl} {"Fs"=1000.0, "#s"=1000.0} ("sampling info"), "Fs"=w576, "#s"=w598) -> (w600:cluster{"Fs":dbl, "#s":dbl})
                          n239 = Bundle By Name(cluster=cluster{"Fs":dbl, "#s":dbl} {"Fs"=1000.0, "#s"=1000.0} ("sampling info"), "Fs"=w576, "#s"=w589) -> (w591:cluster{"Fs":dbl, "#s":dbl})
                          n240 = call <vilib>:"Square Waveform.vi"("duty cycle (%)"=0.0, "offset"=0.0, "sampling info"=w591, "reset signal"=TRUE, "amplitude"=w584, "frequency"=w575) -> ("signal out"=w579:waveform(dbl))  [unwired: 4 in, 1 out]
                          n241 = call <vilib>:"Square Waveform.vi"("duty cycle (%)"=0.0, "offset"=0.0, "sampling info"=w600, "reset signal"=TRUE, "amplitude"=w584, "frequency"=w575) -> ("signal out"=w597:waveform(dbl))  [unwired: 4 in, 1 out]
                          n242 = local read "一个凸起波形图"() -> (w596:dynamicdata)
                          n243 = local read "一个凸起波形图"() -> (w583:dynamicdata)
                          n244 = call "拼接信号11"("Input Signal B"=w596, "Input Signal A"=w597) -> ("Appended Signals"=w582:dynamicdata)  [unwired: 8 in, 1 out]
                          n245 = call "拼接信号12"("Input Signal B"=w583, "Input Signal A"=w579) -> ("Appended Signals"=w581:dynamicdata)  [unwired: 8 in, 1 out]
                          n246 = call "拼接信号10"("Input Signal B"=w581, "Input Signal A"=w582) -> ("Appended Signals"=→"中、短平+2凸":dynamicdata)  [unwired: 8 in, 1 out]
                        }
                        frame #4 {
                          n247 = local read "起始偏移（方波）"() -> (w618:dbl)
                          n248 = Divide(x=w634, y=2.0) -> (x/y=w630:dbl)
                          n249 = Divide(x=w632, y=w633) -> (x/y=w639:dbl)
                          n250 = Greater Or Equal?(x=w608, y=2.0) -> (x >= y?=w613:bool)
                          n251 = Multiply(x=w639, y=w618) -> (x*y=w638:dbl)
                          n252 = case shown="真" w613 {
                            tunnel: [w651 w656] -> w627
                            tunnel: w608 -> [w650 w655]
                            frame False {
                              n253 = case shown="1, 默认" w650 {
                                tunnel: [w652] -> w651
                                frame 1, Default {
                                n254 = local read "中、短平+2凸"() -> (w653:dynamicdata)
                                n255 = local read "起始平+1凸"() -> (w654:dynamicdata)
                                n256 = call "拼接信号4"("Input Signal B"=w653, "Input Signal A"=w654) -> ("Appended Signals"=w652:dynamicdata)  [unwired: 8 in, 1 out]
                                }
                              }
                            }
                            frame True {
                              n257 = stacked-sequence {
                                tunnel: [_ _ w665] -> w656
                                tunnel: w655 -> [_ w659 _]
                                frame #0 {
                                n258 = local read "起始平+1凸"() -> (w657:dynamicdata)
                                n259 = local write "间隔长平+凸信号"(w657) -> ()
                                }
                                frame #1 {
                                n260 = Decrement(x=w659) -> (x-1=w658:dbl)
                                n261 = for {
                                N: w658 -> [_]
                                n262 = local read "间隔长平+凸信号"() -> (w662:dynamicdata)
                                n263 = local read "长平+1凸"() -> (w661:dynamicdata)
                                n264 = call "拼接信号7"("Input Signal B"=w661, "Input Signal A"=w662) -> ("Appended Signals"=w660:dynamicdata)  [unwired: 8 in, 1 out]
                                n265 = local write "间隔长平+凸信号"(w660) -> ()
                                }
                                }
                                frame #2 {
                                n266 = local read "间隔长平+凸信号"() -> (w664:dynamicdata)
                                n267 = local read "中、短平+2凸"() -> (w663:dynamicdata)
                                n268 = call "拼接信号9"("Input Signal B"=w663, "Input Signal A"=w664) -> ("Appended Signals"=w665:dynamicdata)  [unwired: 8 in, 1 out]
                                }
                              }
                            }
                          }
                          n269 = Bundle By Name(cluster=cluster{"Fs":dbl, "#s":dbl} {"Fs"=1000.0, "#s"=1000.0} ("sampling info"), "Fs"=w632, "#s"=w638) -> (w640:cluster{"Fs":dbl, "#s":dbl})
                          n270 = call <vilib>:"Square Waveform.vi"("duty cycle (%)"=0.0, "offset"=0.0, "sampling info"=w640, "reset signal"=TRUE, "amplitude"=w630, "frequency"=w633) -> ("signal out"=w628:waveform(dbl))  [unwired: 4 in, 1 out]
                          n271 = local read "长平+1凸"() -> (w629:dynamicdata)
                          n272 = call "拼接信号14"("Input Signal B"=w628, "Input Signal A"=w629) -> ("Appended Signals"=w625:dynamicdata)  [unwired: 8 in, 1 out]
                          n273 = Subtract(x=w611, y=4.0) -> (x-y=w609:dbl)
                          n274 = Decrement(x=w608) -> (x-1=w607:dbl)
                          n275 = Subtract(x=w609, y=w607) -> (x-y=w603:dbl)
                          n276 = Decrement(x=w603) -> (x-1=w604:dbl)
                          n277 = Greater Or Equal?(x=w603, y=1.0) -> (x >= y?=w605:bool)
                          n278 = case shown="真" w605 {
                            tunnel: w604 -> [_ w643]
                            tunnel: [_ w642] -> w602
                            frame False {
                            }
                            frame True {
                              n279 = stacked-sequence {
                                tunnel: w643 -> [_ w645 _]
                                tunnel: [_ _ w649] -> w642
                                frame #0 {
                                n280 = local read "长平+1凸"() -> (w644:dynamicdata)
                                n281 = local write "长平组信号"(w644) -> ()
                                }
                                frame #1 {
                                n282 = for {
                                N: w645 -> [_]
                                n283 = local read "长平组信号"() -> (w648:dynamicdata)
                                n284 = local read "长平+1凸"() -> (w647:dynamicdata)
                                n285 = call "拼接信号13"("Input Signal B"=w647, "Input Signal A"=w648) -> ("Appended Signals"=w646:dynamicdata)  [unwired: 8 in, 1 out]
                                n286 = local write "长平组信号"(w646) -> ()
                                }
                                }
                                frame #2 {
                                n287 = local read "长平组信号"() -> (w649:dynamicdata)
                                }
                              }
                            }
                          }
                          n288 = call "拼接信号20"("Input Signal B"=w602, "Input Signal A"=w627) -> ("Appended Signals"=w626:dynamicdata)  [unwired: 8 in, 1 out]
                          n289 = call "拼接信号21"("Input Signal B"=w625, "Input Signal A"=w626) -> ("Appended Signals"=w617:dynamicdata)  [unwired: 8 in, 1 out]
                          n290 = case shown="真" w615 {
                            tunnel: w617 -> [w666 w668]
                            tunnel: [w666 w667] -> w616
                            frame False {
                            }
                            frame True {
                              n291 = Negate(x=w668) -> (-x=w667:dynamicdata)
                            }
                          }
                          n292 = Add(x=w630, y=w616) -> (x+y=w624:dynamicdata)
                          n293 = Bundle By Name("Y"=dbl[] []) -> (w621:waveform(dbl))  [unwired: 1 in]
                          n294 = case shown="1, 默认" w612 {
                            tunnel: w624 -> [w670 _]
                            tunnel: [w670 w671] -> w623
                            tunnel: w621 -> [w669 w671]
                            tunnel: [w669 w671] -> w620
                            tunnel: [w669 w671] -> w619
                            frame 1, Default {
                            }
                            frame 0 {
                            }
                          }
                        }
                      }
                    }
                  }
                }
                frame 2 {
                  n295 = Equal?(x=w687, y=1) -> (x = y?=w684:bool)
                  n296 = Equal?(x=w672, y=2) -> (x = y?=w683:bool)
                  n297 = local read "1波形图"() -> (w681:waveform(dbl))
                  n298 = local read "5波形图"() -> (w674:waveform(dbl))
                  n299 = local read "6波形图"() -> (w673:waveform(dbl))
                  n300 = Bundle By Name("Y"=dbl[] []) -> (w678:waveform(dbl))  [unwired: 1 in]
                  n301 = And(x=w684, y=w683) -> (x .and. y?=w682:bool)
                  n302 = case shown="假" w682 {
                    tunnel: w681 -> [_ w709]
                    tunnel: [w688 w709] -> w680
                    tunnel: w678 -> [w692 w708]
                    tunnel: [w690 w708] -> w677
                    tunnel: [w689 w708] -> w676
                    tunnel: w675 -> [w696 _]
                    tunnel: w674 -> [w694 _]
                    tunnel: w673 -> [w693 _]
                    tunnel: w672 -> [w691 _]
                    frame False {
                      n303 = Equal To 0?(x=w696) -> (x = 0?=w695:bool)
                      n304 = case shown="真" w695 {
                        tunnel: w694 -> [_ w698]
                        tunnel: w693 -> [_ w697]
                        tunnel: w692 -> [_ w702]
                        tunnel: w691 -> [_ w703]
                        tunnel: [_ w701] -> w690
                        tunnel: [_ w700] -> w689
                        tunnel: [_ w699] -> w688
                        frame False {
                        }
                        frame True {
                          n305 = case shown="4" w703 {
                            tunnel: [w704 w705] -> w701
                            tunnel: w702 -> [w704 w707]
                            tunnel: [w704 w706] -> w700
                            tunnel: [w704 w707] -> w699
                            tunnel: w698 -> [_ w706]
                            tunnel: w697 -> [_ w705]
                            frame 2, Default {
                            }
                            frame 4 {
                            }
                          }
                        }
                      }
                    }
                    frame True {
                    }
                  }
                }
              }
              "Hall Channel 1" <- w42
              "ME Channel 3" <- w29
              "ME Channel 4" <- w41
              n306 = case shown="0, 默认" w99 {
                tunnel: w101 -> [w724 w1007 _]
                tunnel: "Speed FM" -> [w723 w1008 _]
                tunnel: w98 -> [w722 w1010 _]
                tunnel: "波形发生率Fs" -> [w721 w1009 _]
                tunnel: w97 -> [w720 w1006 _]
                tunnel: [w713 w1005 w1101] -> w27
                tunnel: w94 -> [w719 w1001 _]
                tunnel: w95 -> [w718 _ _]
                tunnel: w96 -> [w717 w1003 _]
                tunnel: w95 -> [w716 w1002 _]
                tunnel: [w715 w1004 w1101] -> w26
                tunnel: [w714 w1000 w1101] -> w43
                tunnel: [w712 w998 0.0] -> w47
                tunnel: w25 -> [w710 w999 _]
                tunnel: w59 -> [w711 _ _]
                frame 0, Default {
                  n307 = stacked-sequence "层叠式顺序结构" {
                    tunnel: w724 -> [w731 _ _ _ w891]
                    tunnel: w723 -> [w725 w760 w789 w835 w893]
                    tunnel: w722 -> [w743 w759 _ w833 w892]
                    tunnel: w721 -> [w730 w761 w790 w836 w894]
                    tunnel: w720 -> [w742 _ _ w834 w889]
                    tunnel: w719 -> [_ w757 w788 w838 w886]
                    tunnel: w718 -> [w729 _ _ _ _]
                    tunnel: w717 -> [_ _ _ _ w888]
                    tunnel: w716 -> [_ _ _ _ _]
                    tunnel: [_ _ _ _ w901] -> w715
                    tunnel: [_ _ _ _ w899] -> w714
                    tunnel: [_ _ _ _ w895] -> w713
                    tunnel: [w726 _ _ _ _] -> w712
                    tunnel: w711 -> [_ _ _ _ w883]
                    tunnel: w710 -> [_ _ _ _ w879]
                    frame #0 {
                      n308 = Equal To 0?(x=w725) -> (x = 0?=w728:bool)
                      n309 = Divide(x=w730, y=w725) -> (x/y=w737:dbl)
                      n310 = case shown="真" w728 {
                        tunnel: w725 -> [w751 _]
                        tunnel: w729 -> [w749 _]
                        tunnel: [w745 0.0] -> w727
                        frame False {
                          n311 = Reciprocal(x=w751) -> (1/x=w750:dbl)
                          n312 = Multiply(x=w749, y=w750) -> (x*y=w748:dbl)
                          n313 = Reciprocal(x=w748) -> (1/x=w747:dbl)
                          n314 = Multiply(x=w747, y=60.0) -> (x*y=w745:dbl)
                        }
                        frame True {
                        }
                      }
                      n315 = Divide(x=w743, y=2.0) -> (x/y=w732:dbl)
                      "曲轴正弦偏移量" <- w732
                      n316 = Multiply(x=w737, y=w731) -> (x*y=w740:dbl)
                      n317 = Bundle By Name(cluster=cluster{"Fs":dbl, "#s":dbl} {"Fs"=1000.0, "#s"=1000.0} ("sampling info"), "Fs"=w730, "#s"=w740) -> (w741:cluster{"Fs":dbl, "#s":dbl})
                      n318 = call <vilib>:"Sine Waveform.vi"("offset"=0.0, "sampling info"=w741, "reset signal"=TRUE, "amplitude"=w732, "frequency"=w725) -> ("signal out"=w739:waveform(dbl))  [unwired: 5 in, 1 out]
                      n319 = case shown="真" w742 {
                        tunnel: w739 -> [w754 w755]
                        tunnel: [w753 w755] -> w738
                        frame False {
                          n320 = Negate(x=w754) -> (-x=w753:waveform(dbl))
                        }
                        frame True {
                        }
                      }
                      n321 = Round To Nearest(number=w727) -> (nearest integer value=w726:dbl)
                      n322 = Add(x=w732, y=w738) -> (x+y=→"曲轴正弦波形图":waveform(dbl))
                    }
                    frame #1 {
                      n323 = Equal To 0?(x=w757) -> (x = 0?=w756:bool)
                      n324 = Not(x=w756) -> (.not. x?=w758:bool)
                      n325 = case shown="真" w758 {
                        tunnel: w761 -> [_ w766]
                        tunnel: w760 -> [_ w765]
                        tunnel: w759 -> [_ w762]
                        frame False {
                        }
                        frame True {
                          n326 = Divide(x=w766, y=w765) -> (x/y=w764:dbl)
                          n327 = Multiply(x=0.4, y=w764) -> (x*y=w769:dbl)
                          n328 = Divide(x=w762, y=2.0) -> (x/y=w763:dbl)
                          n329 = Bundle By Name(cluster=cluster{"Fs":dbl, "#s":dbl} {"Fs"=1000.0, "#s"=1000.0} ("sampling info"), "Fs"=w766, "#s"=w769) -> (w785:cluster{"Fs":dbl, "#s":dbl})
                          n330 = Multiply(x=0.3, y=w764) -> (x*y=w775:dbl)
                          "圆弧点数" <- w775
                          n331 = call <vilib>:"Sine Waveform.vi"("offset"=0.0, "sampling info"=w785, "reset signal"=TRUE, "amplitude"=w763, "frequency"=w765) -> ("signal out"=w780:waveform(dbl))  [unwired: 5 in, 1 out]
                          "部分\n正弦\n波形图" <- w780
                          n332 = To Long Integer(number=w775) -> (32bit integer=w778:i32)
                          n333 = Unbundle By Name(w780) -> ("t0"=→"t0":timestamp, "dt"=→"dt":dbl, "Y"=w781:dbl[])
                          n334 = Increment(x=w778) -> (x+1=→"循环次数":i32)
                          n335 = Array Size(array=w781) -> (size(s)=w783:i32)
                          n336 = Decrement(x=w783) -> (x-1=w782:i32)
                          n337 = Index Array(array=w781, index=w782) -> (element=w776:dbl)
                          "圆半径" <- w776
                          n338 = Divide(x=w776, y=w775) -> (x/y=→"x轴取点间隔":dbl)
                        }
                      }
                    }
                    frame #2 {
                      n339 = Equal To 0?(x=w788) -> (x = 0?=w787:bool)
                      n340 = Not(x=w787) -> (.not. x?=w786:bool)
                      n341 = case shown="真" w786 {
                        tunnel: w790 -> [_ w795]
                        tunnel: w789 -> [_ w794]
                        tunnel: w788 -> [_ w791]
                        frame False {
                        }
                        frame True {
                          n342 = local read "循环次数"() -> (w817:i32)
                          n343 = Increment(x=w791) -> (x+1=w798:dbl)
                          n344 = Divide(x=w798, y=2.0) -> (x/y=w797:dbl)
                          n345 = for {
                            N: w817 -> [_]
                            tunnel: [w828] -> w816 mode=indexing
                            i -> [w829]
                            n346 = local read "x轴取点间隔"() -> (w830:dbl)
                            n347 = Multiply(x=w830, y=w829) -> (x*y=w831:dbl)
                            n348 = Add(x=0.0, y=w831) -> (x+y=w828:dbl)
                          }
                          n349 = Subtract(x=w797, y=0.7) -> (x-y=w792:dbl)
                          n350 = local read "圆半径"() -> (w818:dbl)
                          n351 = Divide(x=w795, y=w794) -> (x/y=w793:dbl)
                          n352 = Multiply(x=w793, y=w792) -> (x*y=w810:dbl)
                          n353 = Multiply(x=2.0, y=w818) -> (x*y=w826:dbl)
                          n354 = Bundle By Name(cluster=cluster{"Fs":dbl, "#s":dbl} {"Fs"=1000.0, "#s"=1000.0} ("sampling info"), "Fs"=w795, "#s"=w810) -> (w811:cluster{"Fs":dbl, "#s":dbl})
                          n355 = Square(x=w816) -> (x^2=w824:dbl[])
                          n356 = Multiply(x=w816, y=w826) -> (x*y=w825:dbl[])
                          n357 = call <vilib>:"Square Waveform.vi"("duty cycle (%)"=0.0, "offset"=0.0, "sampling info"=w811, "reset signal"=TRUE, "amplitude"=0.0, "frequency"=w794) -> ("signal out"=w809:waveform(dbl))  [unwired: 4 in, 1 out]
                          n358 = Subtract(x=w825, y=w824) -> (x-y=w823:dbl[])
                          n359 = Square Root(x=w823) -> (sqrt(x)=w822:dbl[])
                          n360 = Subtract(x=w818, y=w822) -> (x-y=w821:dbl[])
                          n361 = local read "t0"() -> (w808:timestamp)
                          n362 = local read "dt"() -> (w807:dbl)
                          n363 = Bundle By Name("Y"=w809, "t0"=w808, "dt"=w807) -> (w805:waveform(dbl))  [unwired: 1 in]
                          "半\n缺\n齿\n水\n平\n线" <- w805
                          n364 = local read "部分\n正弦\n波形图"() -> (w804:waveform(dbl))
                          n365 = Delete From Array(array=w821, length=1 ("索引"), index=0 ("长度")) -> (array with subset deleted=w815:dbl[])  [unwired: 1 out]
                          n366 = Bundle By Name("Y"=w815, "t0"=w808, "dt"=w807) -> (w806:waveform(dbl))  [unwired: 1 in]
                          "圆\n弧" <- w806
                          n367 = call "拼接信号"("Input Signal B"=w805, "Input Signal A"=w806) -> ("Appended Signals"=w803:dynamicdata)  [unwired: 8 in, 1 out]
                          "圆\n弧\n+\n水\n平" <- w803
                          n368 = call "拼接信号2"("Input Signal B"=w803, "Input Signal A"=w804) -> ("Appended Signals"=→"未\n翻\n转\n半\n缺\n齿":dynamicdata)  [unwired: 8 in, 1 out]
                        }
                      }
                    }
                    frame #3 {
                      n369 = Equal To 0?(x=w838) -> (x = 0?=w837:bool)
                      n370 = Not(x=w837) -> (.not. x?=w839:bool)
                      n371 = case shown="真" w839 {
                        tunnel: [w850 w863] -> w840
                        tunnel: w833 -> [w847 _]
                        tunnel: w836 -> [w846 _]
                        tunnel: w835 -> [w841 _]
                        tunnel: w834 -> [w845 w862]
                        frame False {
                          n372 = Multiply(x=w841, y=2.0) -> (x*y=w843:dbl)
                          n373 = Divide(x=w846, y=w843) -> (x/y=w855:dbl)
                          n374 = Multiply(x=w855, y=2.0) -> (x*y=w857:dbl)
                          n375 = Divide(x=w847, y=2.0) -> (x/y=w848:dbl)
                          n376 = Bundle By Name(cluster=cluster{"Fs":dbl, "#s":dbl} {"Fs"=1000.0, "#s"=1000.0} ("sampling info"), "Fs"=w846, "#s"=w857) -> (w858:cluster{"Fs":dbl, "#s":dbl})
                          n377 = call <vilib>:"Sine Waveform.vi"("offset"=0.0, "sampling info"=w858, "reset signal"=TRUE, "amplitude"=w848, "frequency"=w843) -> ("signal out"=w856:waveform(dbl))  [unwired: 5 in, 1 out]
                          n378 = case shown="真" w845 {
                            tunnel: w856 -> [w860 w861]
                            tunnel: [w859 w861] -> w849
                            frame False {
                              n379 = Negate(x=w860) -> (-x=w859:waveform(dbl))
                            }
                            frame True {
                            }
                          }
                          n380 = Add(x=w848, y=w849) -> (x+y=w850:waveform(dbl))
                        }
                        frame True {
                          n381 = local read "未\n翻\n转\n半\n缺\n齿"() -> (w873:dynamicdata)
                          n382 = call "从动态数据转换"("Dynamic Data Type"=w873) -> ("Array"=w872:dbl[])  [unwired: 3 in]
                          n383 = local read "t0"() -> (w870:timestamp)
                          n384 = local read "dt"() -> (w869:dbl)
                          n385 = Reverse 1D Array(array=w872) -> (reversed array=w871:dbl[])
                          n386 = Negate(x=w872) -> (-x=w874:dbl[])
                          n387 = Bundle By Name("Y"=w871, "t0"=w870, "dt"=w869) -> (w867:waveform(dbl))  [unwired: 1 in]
                          n388 = Bundle By Name("Y"=w874, "t0"=w870, "dt"=w869) -> (w868:waveform(dbl))  [unwired: 1 in]
                          n389 = call "拼接信号3"("Input Signal B"=w867, "Input Signal A"=w868) -> ("Appended Signals"=w865:dynamicdata)  [unwired: 8 in, 1 out]
                          n390 = local read "曲轴正弦偏移量"() -> (w866:dbl)
                          n391 = case shown="假" w862 {
                            tunnel: w865 -> [w875 w877]
                            tunnel: [w875 w876] -> w864
                            frame False {
                            }
                            frame True {
                              n392 = Negate(x=w877) -> (-x=w876:dynamicdata)
                            }
                          }
                          n393 = Add(x=w866, y=w864) -> (x+y=w863:dynamicdata)
                        }
                      }
                      "完\n整\n缺\n齿\n波" <- w840
                    }
                    frame #4 {
                      n394 = local read "曲轴正弦波形图"() -> (w903:waveform(dbl))
                      n395 = Not Equal To 0?(x=w886) -> (x != 0?=w884:bool)
                      n396 = local read "完\n整\n缺\n齿\n波"() -> (w902:waveform(dbl))
                      n397 = Equal?(x=w888, y=4.0) -> (x = y?=w885:bool)
                      n398 = call "曲-缺"("Input Signal B"=w902, "Input Signal A"=w903) -> ("Appended Signals"=w881:dynamicdata)  [unwired: 8 in, 1 out]
                      "曲轴" <- w881
                      n399 = Greater Than 0?(x=w879) -> (x > 0?=w882:bool)
                      n400 = Decrement(x=w879) -> (x-1=w878:dbl)
                      n401 = case shown="真" w885 {
                        tunnel: w894 -> [_ w922]
                        tunnel: w893 -> [_ w921]
                        tunnel: w892 -> [_ w920]
                        tunnel: w891 -> [_ w919]
                        tunnel: [_ w918] -> w890
                        tunnel: w889 -> [_ w917]
                        tunnel: w884 -> [_ w916]
                        tunnel: w881 -> [_ w915]
                        tunnel: w883 -> [_ w914]
                        frame False {
                        }
                        frame True {
                          n402 = case shown="真" w916 {
                            tunnel: w922 -> [_ w934]
                            tunnel: w921 -> [_ w933]
                            tunnel: w920 -> [_ w931]
                            tunnel: w919 -> [_ w929]
                            tunnel: [w923 w928] -> w918
                            tunnel: w917 -> [_ w927]
                            tunnel: w915 -> [w923 _]
                            tunnel: w914 -> [_ w924]
                            frame False {
                            }
                            frame True {
                              n403 = stacked-sequence {
                                tunnel: w934 -> [w943 w965]
                                tunnel: w933 -> [w944 w966]
                                tunnel: [_ w960] -> w932
                                tunnel: w931 -> [w945 w957]
                                tunnel: w929 -> [w942 _]
                                tunnel: w927 -> [w940 w964]
                                tunnel: [_ w959] -> w926
                                tunnel: [w936 _] -> w925
                                tunnel: w924 -> [w935 w956]
                                frame #0 {
                                n404 = Subtract(x=w942, y=w935) -> (x-y=w941:dbl)
                                n405 = Divide(x=w943, y=w944) -> (x/y=w950:dbl)
                                n406 = Multiply(x=w950, y=w941) -> (x*y=w951:dbl)
                                n407 = Divide(x=w945, y=2.0) -> (x/y=w937:dbl)
                                n408 = Bundle By Name(cluster=cluster{"Fs":dbl, "#s":dbl} {"Fs"=1000.0, "#s"=1000.0} ("sampling info"), "Fs"=w943, "#s"=w951) -> (w952:cluster{"Fs":dbl, "#s":dbl})
                                n409 = call <vilib>:"Sine Waveform.vi"("offset"=0.0, "sampling info"=w952, "reset signal"=TRUE, "amplitude"=w937, "frequency"=w944) -> ("signal out"=w939:waveform(dbl))  [unwired: 5 in, 1 out]
                                n410 = case shown="真" w940 {
                                tunnel: w939 -> [w953 w955]
                                tunnel: [w953 w954] -> w938
                                frame False {
                                }
                                frame True {
                                n411 = Negate(x=w955) -> (-x=w954:waveform(dbl))
                                }
                                }
                                n412 = Add(x=w938, y=w937) -> (x+y=w936:waveform(dbl))
                                }
                                frame #1 {
                                n413 = Divide(x=w965, y=w966) -> (x/y=w971:dbl)
                                n414 = Multiply(x=w971, y=w956) -> (x*y=w972:dbl)
                                n415 = Divide(x=w957, y=2.0) -> (x/y=w961:dbl)
                                n416 = local read "完\n整\n缺\n齿\n波"() -> (w958:waveform(dbl))
                                n417 = Bundle By Name(cluster=cluster{"Fs":dbl, "#s":dbl} {"Fs"=1000.0, "#s"=1000.0} ("sampling info"), "Fs"=w965, "#s"=w972) -> (w973:cluster{"Fs":dbl, "#s":dbl})
                                n418 = call <vilib>:"Sine Waveform.vi"("offset"=0.0, "sampling info"=w973, "reset signal"=TRUE, "amplitude"=w961, "frequency"=w966) -> ("signal out"=w963:waveform(dbl))  [unwired: 5 in, 1 out]
                                n419 = case shown="真" w964 {
                                tunnel: w963 -> [w977 w981]
                                tunnel: [w974 w981] -> w962
                                tunnel: [w979 w982] -> w959
                                tunnel: w958 -> [w980 w982]
                                tunnel: w957 -> [w976 _]
                                frame False {
                                n420 = Negate(x=w977) -> (-x=w975:waveform(dbl))
                                n421 = Negate(x=w980) -> (-x=w978:waveform(dbl))
                                n422 = Add(x=w975, y=w976) -> (x+y=w974:waveform(dbl))
                                n423 = Add(x=w976, y=w978) -> (x+y=w979:waveform(dbl))
                                }
                                frame True {
                                }
                                }
                                n424 = Add(x=w962, y=w961) -> (x+y=w960:waveform(dbl))
                                }
                              }
                              n425 = call "拼接信号23"("Input Signal B"=w932, "Input Signal A"=w926) -> ("Appended Signals"=w930:dynamicdata)  [unwired: 8 in, 1 out]
                              n426 = call "拼接信号24"("Input Signal B"=w930, "Input Signal A"=w925) -> ("Appended Signals"=w928:dynamicdata)  [unwired: 8 in, 1 out]
                            }
                          }
                        }
                      }
                      n427 = case shown="真" w882 {
                        tunnel: w881 -> [_ w906]
                        tunnel: [_ w905] -> w880
                        tunnel: w878 -> [_ w904]
                        frame False {
                        }
                        frame True {
                          n428 = stacked-sequence {
                            tunnel: w906 -> [w907 w909 _]
                            tunnel: [_ _ w913] -> w905
                            tunnel: w904 -> [_ w908 _]
                            frame #0 {
                              n429 = local write "曲轴圈数信号"(w907) -> ()
                            }
                            frame #1 {
                              n430 = for {
                                N: w908 -> [_]
                                tunnel: w909 -> [w912]
                                n431 = local read "曲轴圈数信号"() -> (w911:dynamicdata)
                                n432 = call "拼接信号18"("Input Signal B"=w912, "Input Signal A"=w911) -> ("Appended Signals"=w910:dynamicdata)  [unwired: 8 in, 1 out]
                                n433 = local write "曲轴圈数信号"(w910) -> ()
                              }
                            }
                            frame #2 {
                              n434 = local read "曲轴圈数信号"() -> (w913:dynamicdata)
                            }
                          }
                        }
                      }
                      n435 = Bundle By Name("Y"=dbl[] []) -> (w898:waveform(dbl))  [unwired: 1 in]
                      n436 = case shown="4" w888 {
                        tunnel: w880 -> [w984 w988 w995]
                        tunnel: [w984 w988 w992] -> w901
                        tunnel: w892 -> [_ w986 w997]
                        tunnel: [w983 w987 w996] -> w899
                        tunnel: w898 -> [w983 w985 w993]
                        tunnel: [w983 w985 w994] -> w897
                        tunnel: [w983 w985 w995] -> w896
                        tunnel: [w983 w985 w993] -> w895
                        tunnel: w886 -> [_ _ _]
                        tunnel: w890 -> [_ _ w992]
                        frame 1 {
                        }
                        frame 2, Default {
                          n437 = Negate(x=w988) -> (-x=w989:dynamicdata)
                          n438 = Add(x=w989, y=w986) -> (x+y=w987:dynamicdata)
                        }
                        frame 4 {
                          n439 = Negate(x=w992) -> (-x=w991:dynamicdata)
                          n440 = Negate(x=w995) -> (-x=w990:dynamicdata)
                          n441 = Add(x=w997, y=w990) -> (x+y=w994:dynamicdata)
                          n442 = Add(x=w991, y=w997) -> (x+y=w996:dynamicdata)
                        }
                      }
                      "5波形图" <- w897
                      "6波形图" <- w896
                    }
                  }
                }
                frame 1 {
                  n443 = stacked-sequence {
                    tunnel: w1010 -> [w1022 w1038 w1064]
                    tunnel: w1009 -> [w1021 w1052 _]
                    tunnel: w1008 -> [w1015 w1051 _]
                    tunnel: w1007 -> [w1020 _ _]
                    tunnel: w1006 -> [_ _ w1073]
                    tunnel: [_ _ w1070] -> w1005
                    tunnel: [_ _ w1071] -> w1004
                    tunnel: w1003 -> [_ _ w1075]
                    tunnel: w1002 -> [w1013 _ _]
                    tunnel: w1001 -> [_ w1047 _]
                    tunnel: [w1012 _ _] -> w998
                    tunnel: [_ _ w1071] -> w1000
                    tunnel: w999 -> [_ _ w1065]
                    frame #0 {
                      n444 = Equal To 0?(x=w1015) -> (x = 0?=w1014:bool)
                      n445 = Divide(x=w1021, y=w1015) -> (x/y=w1027:dbl)
                      n446 = Multiply(x=w1027, y=w1020) -> (x*y=w1028:dbl)
                      n447 = case shown="假" w1014 {
                        tunnel: w1015 -> [w1036 _]
                        tunnel: w1013 -> [w1034 _]
                        tunnel: [w1030 0.0] -> w1011
                        frame False {
                          n448 = Reciprocal(x=w1036) -> (1/x=w1035:dbl)
                          n449 = Multiply(x=w1034, y=w1035) -> (x*y=w1033:dbl)
                          n450 = Reciprocal(x=w1033) -> (1/x=w1032:dbl)
                          n451 = Multiply(x=w1032, y=60.0) -> (x*y=w1030:dbl)
                        }
                        frame True {
                        }
                      }
                      n452 = Divide(x=w1022, y=2.0) -> (x/y=w1017:dbl)
                      "曲轴方波偏移量" <- w1017
                      n453 = Bundle By Name(cluster=cluster{"Fs":dbl, "#s":dbl} {"Fs"=1000.0, "#s"=1000.0} ("sampling info"), "Fs"=w1021, "#s"=w1028) -> (w1029:cluster{"Fs":dbl, "#s":dbl})
                      n454 = call <vilib>:"Square Waveform.vi"("duty cycle (%)"=50.0, "offset"=0.0, "sampling info"=w1029, "reset signal"=TRUE, "amplitude"=w1017, "frequency"=w1015) -> ("signal out"=w1018:waveform(dbl))  [unwired: 4 in, 1 out]
                      n455 = Add(x=w1017, y=w1018) -> (x+y=→"曲轴方波波形图":waveform(dbl))
                      n456 = Round To Nearest(number=w1011) -> (nearest integer value=w1012:dbl)
                    }
                    frame #1 {
                      n457 = Divide(x=w1052, y=w1051) -> (x/y=w1049:dbl)
                      n458 = Divide(x=w1052, y=w1051) -> (x/y=w1061:dbl)
                      n459 = Multiply(x=w1049, y=w1047) -> (x*y=w1048:dbl)
                      n460 = Multiply(x=w1061, y=0.5) -> (x*y=w1062:dbl)
                      n461 = Bundle By Name(cluster=cluster{"Fs":dbl, "#s":dbl} {"Fs"=1000.0, "#s"=1000.0} ("sampling info"), "Fs"=w1052, "#s"=w1062) -> (w1063:cluster{"Fs":dbl, "#s":dbl})
                      n462 = Bundle By Name(cluster=cluster{"Fs":dbl, "#s":dbl} {"Fs"=1000.0, "#s"=1000.0} ("sampling info"), "Fs"=w1052, "#s"=w1048) -> (w1056:cluster{"Fs":dbl, "#s":dbl})
                      n463 = Divide(x=w1038, y=2.0) -> (x/y=w1040:dbl)
                      n464 = call <vilib>:"Square Waveform.vi"("duty cycle (%)"=50.0, "offset"=w1040, "sampling info"=w1063, "reset signal"=TRUE, "amplitude"=w1040, "frequency"=w1051) -> ("signal out"=w1043:waveform(dbl))  [unwired: 4 in, 1 out]
                      n465 = call <vilib>:"Square Waveform.vi"("duty cycle (%)"=100.0, "offset"=w1038, "sampling info"=w1056, "reset signal"=TRUE, "amplitude"=0.0, "frequency"=w1051) -> ("signal out"=w1042:waveform(dbl))  [unwired: 4 in, 1 out]
                      n466 = Negate(x=w1043) -> (-x=w1041:waveform(dbl))
                      n467 = call "拼接信号15"("Input Signal B"=w1042, "Input Signal A"=w1043) -> ("Appended Signals"=w1046:dynamicdata)  [unwired: 8 in, 1 out]
                      n468 = Add(x=w1038, y=w1041) -> (x+y=w1039:waveform(dbl))
                      n469 = call "拼接信号39"("Input Signal B"=w1039, "Input Signal A"=w1046) -> ("Appended Signals"=→"曲轴方波缺齿波形图":dynamicdata)  [unwired: 8 in, 1 out]
                    }
                    frame #2 {
                      n470 = local read "曲轴方波缺齿波形图"() -> (w1077:dynamicdata)
                      n471 = local read "曲轴方波波形图"() -> (w1078:waveform(dbl))
                      n472 = Greater Than 0?(x=w1065) -> (x > 0?=w1066:bool)
                      n473 = call "拼接信号16"("Input Signal B"=w1077, "Input Signal A"=w1078) -> ("Appended Signals"=w1069:dynamicdata)  [unwired: 8 in, 1 out]
                      n474 = Decrement(x=w1065) -> (x-1=w1068:dbl)
                      n475 = case shown="真" w1066 {
                        tunnel: w1069 -> [_ w1081]
                        tunnel: w1068 -> [_ w1080]
                        tunnel: [_ w1079] -> w1067
                        frame False {
                        }
                        frame True {
                          n476 = stacked-sequence {
                            tunnel: w1081 -> [w1082 w1084 _]
                            tunnel: w1080 -> [_ w1083 _]
                            tunnel: [_ _ w1088] -> w1079
                            frame #0 {
                              n477 = local write "曲轴组合波形"(w1082) -> ()
                            }
                            frame #1 {
                              n478 = for {
                                N: w1083 -> [_]
                                tunnel: w1084 -> [w1086]
                                n479 = local read "曲轴组合波形"() -> (w1087:waveform(dbl))
                                n480 = call "拼接信号17"("Input Signal B"=w1086, "Input Signal A"=w1087) -> ("Appended Signals"=w1085:dynamicdata)  [unwired: 8 in, 1 out]
                                n481 = local write "曲轴组合波形"(w1085) -> ()
                              }
                            }
                            frame #2 {
                              n482 = local read "曲轴组合波形"() -> (w1088:waveform(dbl))
                            }
                          }
                        }
                      }
                      n483 = case shown="真" w1073 {
                        tunnel: w1067 -> [w1089 w1093]
                        tunnel: [w1089 w1091] -> w1072
                        tunnel: w1064 -> [_ w1090]
                        frame False {
                        }
                        frame True {
                          n484 = Negate(x=w1093) -> (-x=w1092:waveform(dbl))
                          n485 = Add(x=w1092, y=w1090) -> (x+y=w1091:waveform(dbl))
                        }
                      }
                      n486 = Bundle By Name("Y"=dbl[] []) -> (w1071:waveform(dbl))  [unwired: 1 in]
                      n487 = case shown="2" w1075 {
                        tunnel: w1072 -> [w1095 w1096]
                        tunnel: [w1095 w1097] -> w1070
                        tunnel: w1064 -> [_ w1098]
                        tunnel: [w1094 w1096] -> w1074
                        tunnel: w1071 -> [w1094 _]
                        frame 1, Default {
                        }
                        frame 2 {
                          n488 = Negate(x=w1096) -> (-x=w1099:waveform(dbl))
                          n489 = Add(x=w1099, y=w1098) -> (x+y=w1097:waveform(dbl))
                        }
                      }
                      "1波形图" <- w1074
                    }
                  }
                }
                frame 2 {
                  n490 = Bundle By Name("Y"=dbl[] []) -> (w1101:waveform(dbl))  [unwired: 1 in]
                }
              }
              "Hall Channel 2" <- w27
              "ME Channel 1" <- w26
              "ME Channel 2" <- w43
              "转速表" <- w47
              n491 = property on="AO2 Channel" class="Ring (严格)"() -> ("Value"=w36:u32)  [unwired: 2 in, 2 out]
              n492 = property on="AO0 Channel" class="Ring (严格)"() -> ("Value"=w46:u32)  [unwired: 2 in, 2 out]
              n493 = property on="AO1 Channel" class="Ring (严格)"() -> ("Value"=w45:u32)  [unwired: 2 in, 2 out]
              n494 = property on="AO3 Channel" class="Ring (严格)"() -> ("Value"=w35:u32)  [unwired: 2 in, 2 out]
              n495 = case shown="5" w35 {
                tunnel: w42 -> [w104 _ _ _ _ _]
                tunnel: [w104 w105 w106 w107 w108 w109] -> w39
                tunnel: w27 -> [_ w105 _ _ _ _]
                tunnel: w43 -> [_ _ _ w107 _ _]
                tunnel: w29 -> [_ _ _ _ w108 _]
                tunnel: w41 -> [_ _ _ _ _ w109]
                tunnel: w26 -> [_ _ w106 _ _ _]
                frame 0 {
                }
                frame 1 {
                }
                frame 2, Default {
                }
                frame 3 {
                }
                frame 4 {
                }
                frame 5 {
                }
              }
              n496 = case shown="5" w36 {
                tunnel: w42 -> [w110 _ _ _ _ _]
                tunnel: [w110 w111 w112 w113 w114 w115] -> w40
                tunnel: w27 -> [_ w111 _ _ _ _]
                tunnel: w43 -> [_ _ _ w113 _ _]
                tunnel: w29 -> [_ _ _ _ w114 _]
                tunnel: w41 -> [_ _ _ _ _ w115]
                tunnel: w26 -> [_ _ w112 _ _ _]
                frame 0 {
                }
                frame 1 {
                }
                frame 2, Default {
                }
                frame 3 {
                }
                frame 4 {
                }
                frame 5 {
                }
              }
              n497 = case shown="2, 默认" w45 {
                tunnel: w42 -> [w122 _ _ _ _ _]
                tunnel: [w122 w123 w124 w125 w126 w127] -> w57
                tunnel: w26 -> [_ _ w124 _ _ _]
                tunnel: w43 -> [_ _ _ w125 _ _]
                tunnel: w29 -> [_ _ _ _ w126 _]
                tunnel: w41 -> [_ _ _ _ _ w127]
                tunnel: w27 -> [_ w123 _ _ _ _]
                frame 0 {
                }
                frame 1 {
                }
                frame 2, Default {
                }
                frame 3 {
                }
                frame 4 {
                }
                frame 5 {
                }
              }
              n498 = case shown="0" w46 {
                tunnel: w42 -> [w128 _ _ _ _ _]
                tunnel: [w128 w129 w130 w131 w132 w133] -> w58
                tunnel: w27 -> [_ w129 _ _ _ _]
                tunnel: w26 -> [_ _ w130 _ _ _]
                tunnel: w43 -> [_ _ _ w131 _ _]
                tunnel: w29 -> [_ _ _ _ w132 _]
                tunnel: w41 -> [_ _ _ _ _ w133]
                frame 0 {
                }
                frame 1 {
                }
                frame 2, Default {
                }
                frame 3 {
                }
                frame 4 {
                }
                frame 5 {
                }
              }
              n499 = call "从动态数据转换9"("Dynamic Data Type"=w58) -> ("Array"=w56:dbl[])  [unwired: 3 in]
              n500 = call "从动态数据转换10"("Dynamic Data Type"=w57) -> ("Array"=w55:dbl[])  [unwired: 3 in]
              n501 = call "从动态数据转换3"("Dynamic Data Type"=w40) -> ("Array"=w38:dbl[])  [unwired: 3 in]
              n502 = call "从动态数据转换4"("Dynamic Data Type"=w39) -> ("Array"=w37:dbl[])  [unwired: 3 in]
              n503 = Array Size(array=w56) -> (size(s)=w31:i32)
              "每通道采样数" <- w31
              n504 = Build Array(w56, w55, w38, w37) -> (w103:dbl[][])
              n505 = call-poly <userlib>:"ArtDAQ_Write.vi"("任务句柄"=w21, "自动开始"=FALSE, "数据"=w103, "错误输入"=w28) -> ("任务句柄"=w51:variant, "错误输出"=w50:errorcluster)  [unwired: 9 in, 1 out]
              n506 = First Call?() -> (First Call?: T/F=w49:bool)
              n507 = case shown="真" w49 {
                tunnel: [w116 w121] -> w54
                tunnel: [w117 w120] -> w53
                tunnel: w51 -> [w117 w119]
                tunnel: w50 -> [w116 w118]
                frame False {
                }
                frame True {
                  n508 = call <userlib>:"ArtDAQ_StartTask.vi"("任务句柄"=w119, "错误输入"=w118) -> ("任务句柄"=w120:variant, "错误输出"=w121:errorcluster)  [unwired: 12 in]
                }
              }
              n509 = call <userlib>:"ArtDAQ_IsTaskDone.vi"("任务句柄"=w53, "错误输入"=w54) -> ("任务句柄"=w23:variant, "错误输出"=w22:errorcluster)  [unwired: 11 in, 1 out]
              n510 = Unbundle By Name(w22) -> ("status"=w34:bool)
              n511 = Or(x=w34, y="Stop") -> (x .or. y?=w32:bool)
            }
            n512 = call-poly <userlib>:"ArtDAQ_Timing.vi"("任务句柄"=w18, "采样模式"=w13, "每通道采样数"=w6, "采样率"="采样速率", "错误输入"=w19) -> ("任务句柄"=w10:variant, "错误输出"=w9:errorcluster)  [unwired: 9 in]
            n513 = feedback-in #1(w9) -> ()
            n514 = feedback-in #2(w10) -> ()
            n515 = call <userlib>:"ArtDAQ_ClearTask.vi"("任务句柄"=w5, "错误输入"=w4) -> ("错误输出"=→"错误输出":errorcluster)  [unwired: 13 in]
          }
          frame "Stop" {
            n516 = One Button Dialog(message="The program has stopped" ("消息")) -> ()  [unwired: 1 in, 1 out]
          }
          frame "Edit" {
            n517 = call-by-ref "?"() -> ("品牌"=w1124:string, "车型"=w1123:string, "曲轴信号类型"=w1105:dbl, "曲轴个数"=w1120:dbl, "曲轴圈数"=w1122:dbl, "曲轴电压幅值"=w1119:dbl, "总齿数"=w1121:dbl, "缺齿数"=w1118:dbl, "缺齿偏移"=w1107:dbl, "曲轴是否取反"=w1106:dbl, "凸轮轴信号类型"=w1109:dbl, "凸轮轴个数"=w1117:dbl, "信号个数"=w1110:dbl, "凸轮轴周期"=w1116:dbl, "凸轮轴电压幅值"=w1115:dbl, "起始偏移"=w1114:dbl, "间隔齿数"=w1113:dbl, "插齿间隔"=w1112:dbl, "凸轮轴是否取反"=w1111:dbl, "OK"=w1108:bool)  [unwired: 9 in, 3 out]
            n518 = Not Equal?(x=w1124, y="") -> (x != y?=w1129:bool)
            n519 = And(x=w1108, y=w1129) -> (x .and. y?=w1126:bool)
            n520 = Not Equal?(x=w1123, y="") -> (x != y?=w1127:bool)
            n521 = And(x=w1126, y=w1127) -> (x .and. y?=w1125:bool)
            "数值合法" <- w1125
            n522 = case shown="假" w1125 {
              tunnel: w1124 -> [w1133 w1162]
              tunnel: w1123 -> [w1132 w1161]
              tunnel: w1120 -> [_ w1160]
              tunnel: w1105 -> [_ w1159]
              tunnel: w1122 -> [_ w1158]
              tunnel: w1121 -> [_ w1157]
              tunnel: w1107 -> [_ w1156]
              tunnel: w1119 -> [_ w1155]
              tunnel: w1118 -> [_ w1154]
              tunnel: w1106 -> [_ w1153]
              tunnel: w1117 -> [_ w1152]
              tunnel: w1116 -> [_ w1151]
              tunnel: w1115 -> [_ w1150]
              tunnel: w1114 -> [_ w1149]
              tunnel: w1113 -> [_ w1148]
              tunnel: w1112 -> [_ w1147]
              tunnel: w1111 -> [_ w1146]
              tunnel: w1110 -> [_ w1145]
              tunnel: w1109 -> [_ w1144]
              tunnel: w1108 -> [w1131 _]
              frame False {
                n523 = Equal?(x=w1133, y="") -> (x = y?=w1135:bool)
                n524 = Equal?(x=w1132, y="") -> (x = y?=w1136:bool)
                n525 = And(x=w1131, y=w1135) -> (x .and. y?=w1134:bool)
                n526 = case shown="真" w1134 {
                  tunnel: w1136 -> [w1141 _]
                  tunnel: w1131 -> [w1139 _]
                  frame False {
                    n527 = And(x=w1139, y=w1141) -> (x .and. y?=w1140:bool)
                    n528 = case shown="假" w1140 {
                      frame False {
                      }
                      frame True {
                        n529 = One Button Dialog(message="The model cannot be empty" ("消息")) -> ()  [unwired: 1 in, 1 out]
                      }
                    }
                  }
                  frame True {
                    n530 = One Button Dialog(message="The brand cannot be empty" ("消息")) -> ()  [unwired: 1 in, 1 out]
                  }
                }
              }
              frame True {
                n531 = stacked-sequence {
                  tunnel: w1162 -> [w1165 _ _]
                  tunnel: w1161 -> [w1164 _ _]
                  tunnel: w1160 -> [_ w1173 _]
                  tunnel: w1159 -> [_ w1172 _]
                  tunnel: w1158 -> [_ w1171 _]
                  tunnel: w1157 -> [_ w1167 _]
                  tunnel: w1156 -> [_ w1170 _]
                  tunnel: w1155 -> [_ w1169 _]
                  tunnel: w1154 -> [_ w1168 _]
                  tunnel: w1153 -> [_ w1166 _]
                  tunnel: w1152 -> [_ _ w1202]
                  tunnel: w1151 -> [_ _ w1201]
                  tunnel: w1150 -> [_ _ w1200]
                  tunnel: w1149 -> [_ _ w1199]
                  tunnel: w1148 -> [_ _ w1198]
                  tunnel: w1147 -> [_ _ w1197]
                  tunnel: w1146 -> [_ _ w1196]
                  tunnel: w1145 -> [_ _ w1195]
                  tunnel: w1144 -> [_ _ w1194]
                  frame #0 {
                    n532 = Build Array(w1165, w1164) -> (→"品牌车型数组":string[])
                  }
                  frame #1 {
                    n533 = stacked-sequence {
                      tunnel: w1166 -> [w1182 _]
                      tunnel: w1171 -> [w1180 _]
                      tunnel: w1169 -> [w1179 _]
                      tunnel: w1167 -> [w1178 _]
                      tunnel: w1168 -> [w1177 _]
                      tunnel: w1170 -> [w1176 _]
                      tunnel: w1173 -> [w1175 _]
                      tunnel: w1172 -> [w1174 _]
                      frame #0 {
                        n534 = case shown="1" w1182 {
                          tunnel: [FALSE TRUE] -> w1181
                          frame 0, Default {
                          }
                          frame 1 {
                          }
                        }
                        "0曲轴是否取反" <- w1181
                        "0曲轴轴信号类型" <- w1174
                        "0曲轴电压幅值" <- w1179
                        "0总齿数" <- w1178
                        "0曲轴个数" <- w1175
                        "0缺齿数" <- w1177
                        "0曲轴圈数" <- w1180
                        "0缺齿偏移" <- w1176
                      }
                      frame #1 {
                        n535 = local read "0曲轴轴信号类型"() -> (w1186:u32)
                        n536 = local read "0曲轴圈数"() -> (w1192:dbl)
                        n537 = local read "0缺齿偏移"() -> (w1193:dbl)
                        n538 = local read "0曲轴电压幅值"() -> (w1187:dbl)
                        n539 = local read "0总齿数"() -> (w1188:dbl)
                        n540 = local read "0曲轴个数"() -> (w1189:dbl)
                        n541 = local read "0曲轴是否取反"() -> (w1190:bool)
                        n542 = local read "0缺齿数"() -> (w1191:dbl)
                        n543 = Bundle("0曲轴轴信号类型"=w1186, "0曲轴电压幅值"=w1187, "0总齿数"=w1188, "0曲轴个数"=w1189, "0曲轴是否取反"=w1190, "0缺齿数"=w1191, "0曲轴圈数"=w1192, "0缺齿偏移"=w1193) -> (→"曲轴参数":T5)  [unwired: 1 in]
                      }
                    }
                  }
                  frame #2 {
                    n544 = stacked-sequence {
                      tunnel: w1201 -> [w1212 _]
                      tunnel: w1200 -> [w1211 _]
                      tunnel: w1199 -> [w1210 _]
                      tunnel: w1198 -> [w1209 _]
                      tunnel: w1197 -> [w1208 _]
                      tunnel: w1196 -> [w1207 _]
                      tunnel: w1195 -> [w1205 _]
                      tunnel: w1194 -> [w1204 _]
                      tunnel: w1202 -> [w1203 _]
                      frame #0 {
                        n545 = case shown="1" w1207 {
                          tunnel: [FALSE TRUE] -> w1206
                          frame 0, Default {
                          }
                          frame 1 {
                          }
                        }
                        "0凸轮轴是否取反" <- w1206
                        "0凸轮轴信号类型" <- w1204
                        "0凸轮轴电压幅值" <- w1211
                        "0信号个数" <- w1205
                        "0凸轮轴个数" <- w1203
                        "0凸轮轴周期" <- w1212
                        "0起始偏移" <- w1210
                        "0插齿间隔" <- w1208
                        "0间隔齿数" <- w1209
                      }
                      frame #1 {
                        n546 = local read "0凸轮轴信号类型"() -> (w1216:u32)
                        n547 = local read "0凸轮轴电压幅值"() -> (w1217:dbl)
                        n548 = local read "0信号个数"() -> (w1218:dbl)
                        n549 = local read "0凸轮轴个数"() -> (w1219:dbl)
                        n550 = local read "0凸轮轴是否取反"() -> (w1220:bool)
                        n551 = local read "0凸轮轴周期"() -> (w1221:dbl)
                        n552 = local read "0起始偏移"() -> (w1222:dbl)
                        n553 = local read "0插齿间隔"() -> (w1223:dbl)
                        n554 = local read "0间隔齿数"() -> (w1224:dbl)
                        n555 = Bundle("0凸轮轴信号类型"=w1216, "0凸轮轴电压幅值"=w1217, "0信号个数"=w1218, "0凸轮轴个数"=w1219, "0凸轮轴是否取反"=w1220, "0凸轮轴周期"=w1221, "0起始偏移"=w1222, "0插齿间隔"=w1223, "0间隔齿数"=w1224) -> (→"凸轮轴参数":T2)  [unwired: 1 in]
                      }
                    }
                  }
                }
              }
            }
          }
          frame "Save" {
            n556 = local read "数值合法"() -> (w1229:bool)
            n557 = Equal?(x=w1225, y="保存") -> (x = y?=w1226:bool)
            n558 = And(x=w1226, y=w1229) -> (x .and. y?=w1228:bool)
            n559 = case shown="假" w1228 {
              frame False {
                n560 = One Button Dialog(message="No signal parameters were edited!" ("消息")) -> ()  [unwired: 1 in, 1 out]
              }
              frame True {
                n561 = stacked-sequence {
                  frame #0 {
                    n562 = stacked-sequence {
                      frame #0 {
                        n563 = local read "品牌车型数组"() -> (w1234:string[])
                        n564 = Index Array(array=w1234, index=0 ("索引")) -> (element=w1237:string)
                        "品牌" <- w1237
                        n565 = Index Array(array=w1234, index=1 ("索引")) -> (element=w1233:string)
                        n566 = Current VI's Path() -> (path=w1244:path)
                        n567 = Strip Path(path=w1244) -> (stripped path=w1243:path)  [unwired: 1 out]
                        n568 = Build Path(base path=w1243, name or relative path="品牌文件" ("名称或相对路径")) -> (appended path=w1239:path)
                        n569 = Concatenate Strings(w1237, ".xml") -> (w1240:string)
                        n570 = Build Array(w1233) -> (w1232:string[])
                        "车型数组" <- w1232
                        n571 = Build Path(base path=w1239, name or relative path=w1240) -> (appended path=w1238:path)
                        n572 = Flatten To XML(6:w1232) -> (2:w1231:string)
                        n573 = call-poly <vilib>:"Write to XML File.vi"("Standalone? (T)"=TRUE, "XML Encoding"="GB2312", "XML Input"=w1231, "XML File Path"=w1238) -> ()  [unwired: 5 in, 3 out]
                      }
                      frame #1 {
                        n574 = stacked-sequence {
                          frame #0 {
                            n575 = Current VI's Path() -> (path=w1258:path)
                            n576 = Strip Path(path=w1258) -> (stripped path=w1257:path)  [unwired: 1 out]
                            n577 = Build Path(base path=w1257, name or relative path="品牌文件" ("名称或相对路径")) -> (appended path=w1252:path)
                            n578 = Concatenate Strings("品牌" ("字符串"), ".xml") -> (w1251:string)
                            n579 = Build Path(base path=w1252, name or relative path=w1251) -> (appended path=w1250:path)
                            n580 = call-poly <vilib>:"Read From XML File.vi"("error in (no error)"="error", "XML File Path"=w1250) -> ("error out"=w1260:errorcluster, "XML Elements"=w1259:string)  [unwired: 7 in, 1 out]
                            n581 = Unflatten From XML(xml string=w1259, type="字符串数组类型", error in (no error)=w1260) -> (value=w1248:string[])  [unwired: 1 out]
                            "品牌数组" <- w1248
                            n582 = Array Size(array=w1248) -> (size(s)=→"数组大小":i32)
                          }
                          frame #1 {
                            n583 = local read "品牌数组"() -> (w1263:string[])
                            n584 = local read "品牌"() -> (w1264:string)
                            n585 = local read "数组大小"() -> (w1262:i32)
                            n586 = Insert Into Array(array=w1263, index=w1262, new element=w1264) -> (w1261:string[])
                            n587 = local write "品牌数组"(w1261) -> ()
                          }
                          frame #2 {
                            n588 = Current VI's Path() -> (path=w1275:path)
                            n589 = Strip Path(path=w1275) -> (stripped path=w1274:path)  [unwired: 1 out]
                            n590 = Build Path(base path=w1274, name or relative path="品牌文件" ("名称或相对路径")) -> (appended path=w1270:path)
                            n591 = Concatenate Strings("品牌", ".xml") -> (w1271:string)
                            n592 = local read "品牌数组"() -> (w1266:string[])
                            n593 = Build Path(base path=w1270, name or relative path=w1271) -> (appended path=w1269:path)
                            n594 = Flatten To XML(6:w1266) -> (2:w1265:string)
                            n595 = call-poly <vilib>:"Write to XML File.vi"("Standalone? (T)"=TRUE, "XML Encoding"="GB2312", "XML Input"=w1265, "XML File Path"=w1269) -> ()  [unwired: 5 in, 3 out]
                          }
                        }
                      }
                    }
                  }
                  frame #1 {
                    w1290 = "Camshaft_Signal" ("section")
                    w1336 = "Crank_Signal" ("section")
                    n596 = local read "曲轴参数"() -> (w1367:T3)
                    n597 = local read "凸轮轴参数"() -> (w1318:T2)
                    n598 = Current VI's Path() -> (path=w1333:path)
                    n599 = Unbundle(w1367) -> ("0曲轴轴信号类型"=w1364:u32, "0曲轴电压幅值"=w1362:dbl, "0总齿数"=w1361:dbl, "0曲轴个数"=w1360:dbl, "0曲轴是否取反"=w1363:bool, "0却齿数"=w1365:dbl, "0曲轴圈数"=w1366:dbl, "0缺齿偏移"=w1277:dbl)
                    n600 = Strip Path(path=w1333) -> (stripped path=w1332:path)  [unwired: 1 out]
                    n601 = Unbundle(w1318) -> ("0凸轮轴信号类型"=w1310:u32, "0凸轮轴电压幅值"=w1316:dbl, "0信号个数"=w1311:dbl, "0凸轮轴个数"=w1309:dbl, "0凸轮轴是否取反"=w1312:bool, "0凸轮轴周期"=w1317:dbl, "0起始偏移"=w1315:dbl, "0插齿间隔"=w1313:dbl, "0间隔齿数"=w1314:dbl)
                    n602 = local read "品牌车型数组"() -> (w1323:string[])
                    n603 = Index Array(array=w1323, index=1 ("索引")) -> (element=w1324:string)
                    n604 = Index Array(array=w1323, index=0 ("索引")) -> (element=w1326:string)
                    n605 = Build Path(base path=w1332, name or relative path="曲轴凸轮轴配置文件" ("名称或相对路径")) -> (appended path=w1330:path)
                    n606 = Concatenate Strings(w1324, ".ini" ("字符串")) -> (w1328:string)
                    n607 = Build Path(base path=w1330, name or relative path=w1326) -> (appended path=w1321:path)
                    n608 = String To Path(string=w1328) -> (path=w1322:path)
                    n609 = Create Folder(path (use dialog)=w1321) -> (created path=w1319:path)  [unwired: 2 in, 2 out]
                    n610 = Build Path(base path=w1319, name or relative path=w1322) -> (appended path=w1320:path)
                    n611 = call <vilib>:"Open Config Data.vi"("create file if necessary (T)"=TRUE ("create file if necessary? (T)"), "configuration file path"=w1320) -> ("error out"=w1356:errorcluster, "refnum"=w1354:T4)  [unwired: 7 in, 1 out]
                    n612 = call-poly <vilib>:"Write Key.vi"("section"=w1336, "error in (no error)"=w1356, "value"=w1364, "key"="type", "refnum"=w1354) -> ("error out"=w1357:errorcluster, "refnum out"=w1355:T4)  [unwired: 4 in, 1 out]
                    n613 = call-poly <vilib>:"Write Key.vi"("section"=w1336, "error in (no error)"=w1357, "value"=w1362, "key"="voltage" ("键2"), "refnum"=w1355) -> ("error out"=w1352:errorcluster, "refnum out"=w1351:T4)  [unwired: 4 in, 1 out]
                    n614 = call-poly <vilib>:"Write Key.vi"("section"=w1336, "error in (no error)"=w1352, "value"=w1363, "key"="invert" ("键3"), "refnum"=w1351) -> ("error out"=w1349:errorcluster, "refnum out"=w1348:T4)  [unwired: 4 in, 1 out]
                    n615 = call-poly <vilib>:"Write Key.vi"("section"=w1336, "error in (no error)"=w1349, "value"=w1360, "key"="crank_number" ("键3"), "refnum"=w1348) -> ("error out"=w1346:errorcluster, "refnum out"=w1345:T4)  [unwired: 4 in, 1 out]
                    n616 = call-poly <vilib>:"Write Key.vi"("section"=w1336, "error in (no error)"=w1346, "value"=w1361, "key"="tooth_number" ("键3"), "refnum"=w1345) -> ("error out"=w1343:errorcluster, "refnum out"=w1344:T4)  [unwired: 4 in, 1 out]
                    n617 = call-poly <vilib>:"Write Key.vi"("section"=w1336, "error in (no error)"=w1343, "value"=w1365, "key"="edentulous_number" ("键3"), "refnum"=w1344) -> ("error out"=w1340:errorcluster, "refnum out"=w1339:T4)  [unwired: 4 in, 1 out]
                    n618 = call-poly <vilib>:"Write Key.vi"("section"=w1336, "error in (no error)"=w1340, "value"=w1366, "key"="cylinder_number" ("键3"), "refnum"=w1339) -> ("error out"=w1335:errorcluster, "refnum out"=w1337:T4)  [unwired: 4 in, 1 out]
                    n619 = call-poly <vilib>:"Write Key.vi"("section"=w1336, "error in (no error)"=w1335, "value"=w1277, "key"="edentulous_offset" ("键2"), "refnum"=w1337) -> ("error out"=w1279:errorcluster, "refnum out"=w1280:T4)  [unwired: 4 in, 1 out]
                    n620 = call-poly <vilib>:"Write Key.vi"("section"=w1290, "error in (no error)"=w1279, "value"=w1310, "key"="type" ("键3"), "refnum"=w1280) -> ("error out"=w1308:errorcluster, "refnum out"=w1307:T4)  [unwired: 4 in, 1 out]
                    n621 = call-poly <vilib>:"Write Key.vi"("section"=w1290, "error in (no error)"=w1308, "value"=w1316, "key"="voltage" ("键3"), "refnum"=w1307) -> ("error out"=w1305:errorcluster, "refnum out"=w1303:T4)  [unwired: 4 in, 1 out]
                    n622 = call-poly <vilib>:"Write Key.vi"("section"=w1290, "error in (no error)"=w1305, "value"=w1311, "key"="signal_number" ("键3"), "refnum"=w1303) -> ("error out"=w1299:errorcluster, "refnum out"=w1302:T4)  [unwired: 4 in, 1 out]
                    n623 = call-poly <vilib>:"Write Key.vi"("section"=w1290, "error in (no error)"=w1299, "value"=w1309, "key"="camshaft_number" ("键3"), "refnum"=w1302) -> ("error out"=w1304:errorcluster, "refnum out"=w1301:T4)  [unwired: 4 in, 1 out]
                    n624 = call-poly <vilib>:"Write Key.vi"("section"=w1290, "error in (no error)"=w1304, "value"=w1312, "key"="invert" ("键2"), "refnum"=w1301) -> ("error out"=w1306:errorcluster, "refnum out"=w1300:T4)  [unwired: 4 in, 1 out]
                    n625 = call-poly <vilib>:"Write Key.vi"("section"=w1290, "error in (no error)"=w1306, "value"=w1317, "key"="cycle", "refnum"=w1300) -> ("error out"=w1295:errorcluster, "refnum out"=w1298:T4)  [unwired: 4 in, 1 out]
                    n626 = call-poly <vilib>:"Write Key.vi"("section"=w1290, "error in (no error)"=w1295, "value"=w1315, "key"="start_offset" ("键2"), "refnum"=w1298) -> ("error out"=w1296:errorcluster, "refnum out"=w1297:T4)  [unwired: 4 in, 1 out]
                    n627 = call-poly <vilib>:"Write Key.vi"("section"=w1290, "error in (no error)"=w1296, "value"=w1313, "key"="interpolated_interval", "refnum"=w1297) -> ("error out"=w1293:errorcluster, "refnum out"=w1294:T4)  [unwired: 4 in, 1 out]
                    n628 = call-poly <vilib>:"Write Key.vi"("section"=w1290, "error in (no error)"=w1293, "value"=w1314, "key"="interval_tooth_number", "refnum"=w1294) -> ("error out"=w1292:errorcluster, "refnum out"=w1291:T4)  [unwired: 4 in, 1 out]
                    n629 = call <vilib>:"Close Config Data.vi"("error in (no error)"=w1292, "write file if changed (T)"=TRUE ("write configuration file? (T)"), "refnum"=w1291) -> ()  [unwired: 9 out]
                  }
                  frame #2 {
                    n630 = property on="曲轴参数" class="Clust (严格)"() -> ("DefVal"=w1368:T3)  [unwired: 2 in, 2 out]
                    n631 = property on="凸轮轴参数" class="Clust (严格)"() -> ("DefVal"=w1369:T2)  [unwired: 2 in, 2 out]
                    n632 = property on="品牌车型数组" class="Arr (严格)"() -> ("DefVal"=w1370:string[])  [unwired: 2 in, 2 out]
                    n633 = local write "曲轴参数"(w1368) -> ()
                    n634 = local write "凸轮轴参数"(w1369) -> ()
                    n635 = local write "品牌车型数组"(w1370) -> ()
                  }
                  frame #3 {
                    n636 = One Button Dialog(message="Save success！" ("消息")) -> ()  [unwired: 1 in, 1 out]
                  }
                }
              }
            }
          }
        }
      }
    }
  }
